vi "trancon-main.vi"() -> ()   [LabVIEW 2015]
uses:
  controls/mylistbox.ctl
  controls/radiobuttons-detection.ctl
  controls/radiobuttons-exp.ctl
  controls/graph.ctl
  dependecies/Error Code Enum typedef.ctl
  controls/clustercontrols-measerument.ctl
  Classes/Experiment.lvclass
  <vilib>/DAQmx/write.llb/DAQmx Write (Digital Bool 1Line 1Point).vi
  <vilib>/DAQmx/read.llb/DAQmx Read (Analog 1D DBL 1Chan NSamp).vi
  <vilib>/Analysis/baseanly.llb/Mean (DBL).vi
  <vilib>/DAQmx/read.llb/DAQmx Read (Digital Bool 1Line 1Point).vi
  dependecies/globalVarSD.vi
  <vilib>/DAQmx/miscellaneous.llb/DAQmx Fill In Error Info.vi
  Classes/Experiments_group.lvclass
  <vilib>/Analysis/NI_AALBase.lvlib
panel:
  in  "Relay key":bool
  in  "Statistics":bool
  in  "shift":i32
  in  "Old/New":bool
  in  "Cut On/off":bool
  in  "pixel-":i32=50
  in  "pixel+":i32=450
  out "moved":string
  in  "Delay (mm) 2":i32 min=-700 max=100
  out "Delay (mm)":dbl
  out "Delay (ps)":dbl=-0.0
  in  "type of movement":u16(ring)=2 items=["definir position", "deplacer relatif", "deplacer absolu"]
  out "deplacement boolean":bool
  in  "Move delay line":bool
  out "Initialisation finie":bool
  in  "STOP":bool
  in  "Work/Dev":bool=TRUE
  in  "Experiment type":T1
  in  "Detection type":T2=enum."UV-vis detection"
  in  "Block accelerator":bool=TRUE
  in  "Block laser beam":bool=TRUE
  in  "Move target":bool
  in  "cellule":u16(ring)=1 items=["Cell1", "Cell2", "Cell stat", "Cell3", "Cell4", "Lanex"]
  out "Cell in place":bool
  in  "Slide":i32(slide)=2 scale=0.0..5.0
  in  "Base path":path=path "G:/SD/DATA"
  out "ALARM":bool
  in  "MainTab":enum32{"Real time", "Measurement", "Settings"}(tab)
  in  "Save SC":bool
  in  "# par point":i32=10 min=1 max=100 step=1
  in  "Real time":bool
  in  "Time, ms":dbl=10.0 min=1.0 max=150.0
  in  "Move Crystall":bool
  out "Réglage TR SC":cluster{"Y":dbl[], "Y":dbl[]}[](graph)=[{"Y"=array[512 elements], "Y"=array[512 elements]}, {"Y"=array[512 elements], "Y"=[6.8, 6.2, 16.4, 11.8, 0.8, 9.8, 11.4, 13.6, 13.0, 10.6, 14.2, 8.6, 15.8, 11.0, 8.6, 12.6, 9.6, 9.4, 16.2, 10.8, 15.6, 11.4, 8.8, 13.6, 10.0, 8.2, 14.8, 17.4, 12.8, 13.2, 18.2, 11.8, 12.8, 17.4, 14.8, 19.4, 21.8, 26.4, 26.6, 35.4, 41.6, 41.0, 55.6, 60.6, 73.0, 85.8, 88.0, 106.6, 125.0, 140.0, 168.6, 188.2, 209.0, 235.2, 267.4, 292.2, 320.8, 351.4, 397.6, 431.8, 475.6, 521.0, 576.2, 623.4, 695.8, 752.0, 833.4, 903.2, 1007.2, 1082.6, 1193.2, 1304.0, 1415.6, 1527.0, 1680.0, 1805.8, 1954.8, 2073.4, 2241.6, 2394.8, 2581.2, 2714.2, 2872.8, 3013.0, 3213.8, 3372.8, 3558.2, 3709.8, 3899.4, 4049.0, 4210.8, 4323.8, 4455.6, 4530.8, 4649.8, 4744.0, 4794.6, 4841.8, 4903.0, 4937.2, 4955.8, 4944.6, 5001.2, 5011.4, 4971.0, 4967.4, 4940.8, 4908.2, 4897.6, 4815.8, 4755.8, 4671.6, 4553.6, 4440.2, 4394.8, 4223.6, 4120.6, 3977.6, 3895.6, 3809.4, 3721.6, 3619.8, 3558.4, 3527.6, 3463.8, 3348.6, 3322.4, 3214.2, 3202.0, 3114.2, 3081.6, 3028.0, 2942.6, 2856.0, 2795.8, 2690.2, 2625.4, 2535.4, 2475.2, 2386.8, 2354.8, 2281.4, 2260.0, 2195.0, 2173.0, 2124.6, 2136.8, 2111.2, 2133.2, 2114.2, 2129.8, 2116.8, 2125.0, 2109.8, 2128.6, 2121.6, 2119.8, 2121.2, 2122.4, 2093.8, 2053.0, 1998.8, 1993.8, 1951.4, 1922.2, 1874.6, 1854.2, 1819.4, 1814.0, 1789.8, 1818.2, 1826.6, 1872.8, 1897.4, 2010.0, 2048.2, 2125.8, 2138.2, 2201.8, 2220.2, 2249.8, 2255.6, 2238.8, 2188.8, 2164.8, 2103.4, 2020.4, 1918.8, 1836.0, 1712.0, 1602.4, 1516.4, 1454.8, 1355.2, 1259.0, 1217.8, 1176.2, 1109.6, 1119.4, 1105.2, 1125.6, 1167.2, 1260.4, 1364.4, 1490.8, 1615.0, 1791.8, 1904.0, 2039.4, 2136.6, 2245.0, 2243.6, 2354.2, 2386.6, 2434.0, 2424.0, 2440.2, 2390.0, 2371.8, 2304.0, 2249.2, 2138.0, 2070.4, 1940.8, 1837.6, 1741.6, 1637.4, 1525.2, 1440.2, 1337.4, 1259.6, 1161.8, 1088.6, 1018.8, 954.0, 895.0, 853.2, 793.6, 761.8, 714.4, 693.0, 644.2, 621.8, 580.4, 565.4, 540.6, 521.2, 499.0, 488.4, 464.2, 453.6, 433.0, 425.2, 413.0, 414.4, 391.6, 388.6, 366.0, 368.0, 342.2, 337.4, 316.2, 303.6, 290.2, 278.4, 267.8, 258.4, 241.8, 240.0, 220.2, 221.4, 192.2, 187.2, 167.6, 154.6, 144.6, 137.8, 131.2, 123.4, 107.2, 114.4, 98.0, 98.8, 88.0, 81.0, 75.6, 82.8, 78.0, 72.0, 65.2, 67.4, 62.4, 65.2, 62.0, 60.0, 52.6, 50.2, 47.6, 49.4, 40.6, 45.4, 40.8, 47.4, 41.2, 49.6, 39.0, 42.4, 32.4, 33.4, 32.8, 32.6, 32.4, 35.2, 33.8, 33.8, 33.2, 34.4, 29.2, 33.0, 31.0, 35.4, 28.2, 30.4, 32.6, 27.4, 29.0, 33.8, 33.0, 38.6, 30.0, 34.2, 31.8, 40.0, 33.8, 38.4, 32.0, 38.0, 34.0, 38.4, 31.8, 33.2, 30.6, 34.8, 34.2, 34.8, 25.6, 33.6, 27.8, 36.8, 31.4, 31.2, 28.2, 36.2, 30.6, 27.2, 29.2, 18.0, 20.6, 25.2, 25.2, 21.0, 24.8, 27.0, 23.8, 28.8, 16.2, 26.4, 18.8, 21.8, 16.4, 14.8, 12.0, 18.0, 20.8, 18.2, 10.4, 18.8, 18.4, 15.8, 17.8, 19.2, 16.6, 13.8, 13.4, 16.0, 16.8, 18.2, 15.2, 13.4, 13.8, 16.4, 12.2, 16.0, 14.2, 16.4, 12.2, 21.4, 10.8, 20.0, 12.4, 19.0, 13.8, 23.2, 12.8, 10.2, 12.0, 8.4, 8.6, 19.0, 11.6, 28.4, 11.8, 12.8, 13.8, 14.4, 10.8, 12.0, 6.6, 12.2, 11.2, 18.0, 15.4, 21.8, 10.2, 15.2, 10.4, 10.6, 5.0, 8.6, 7.6, 9.8, 7.4, 13.2, 10.6, 15.2, 7.8, 13.4, 12.6, 15.8, 11.6, 12.6, 9.6, 12.6, 12.2, 15.8, 6.2, 14.2, 12.8, 15.6, 7.0, 12.0, 12.8, 15.8, 10.4, 16.2, 11.6, 18.2, 13.0, 12.8, 6.2, 21.4, 9.2, 11.6, 6.0, 8.0, 6.0, 10.6, 6.0, 14.4, 4.8, 10.4, 9.0, 14.0, 11.0, 11.6, 9.2, 11.4, 4.2, 7.2, 5.8, 11.2, 8.2, 11.0, 8.0, 10.2, 5.6, 9.6, 3.6, 12.2, 6.4, 8.2, 4.2, 4.2, 4.0, 2.6, 9.0, 7.0, 5.6, 8.0, 4.6, 11.2, 4.8, 7.8, 3.4, 6.8, 6.8, 9.2, 7.4, 0.4, 5.0, -1.2, 0.0]}, {"Y"=array[512 elements], "Y"=array[512 elements]}, {"Y"=array[512 elements], "Y"=array[512 elements]}]
  out "Réglage TR OD":T3(graph)
  in  "wavelength fix":dbl=640.0 caption="wave fix"
  in  "ODmax":dbl=1.0
  in  "ODmin":dbl=-1.0
  in  "# par point":i32=15 min=1 max=100 step=1
  out "# current":i32
  out "RDT, ps":dbl=3790.0
  out "Real time exp":T4
  in  "sigma":dbl=1.4 min=0.0 step=0.1
  in  "Clean":bool
  in  "load Exp":bool
  in  "BG correct":bool
  in  "Save":bool
  in  "del exp":bool
  in  "del group":bool
  in  "add exp":bool
  in  "add group":bool
  in  "All":bool
  in  "Average exp":bool
  in  "clean mode":enum32{"delete", "approximate"}(radio)=enum."approximate"
  in  "Commentaires exp":string="...Write experiment description..."
  in  "Commentaires group":string="...write group description..."
  in  "Experiment":T5
  in  "group":u16(ring) items=["1. Init exp", "2. 120417"]
  in  "LogY":bool
  in  "sel kin":i32
  in  "Avr kinetics":bool
  in  "Del kinetics":bool
  in  "Add kinetics":bool
  in  "To Wave":dbl
  in  "From Wave":dbl
  out "Kinetics":cluster{"Y":dbl[], "Y":dbl[]}[](graph)
  in  "DelaysTab":enum32{"Mode Normale", "Table"}(tab)
  in  "Fix":bool=TRUE
  in  "Break measurement":bool
  in  "# points":i32=1 min=1 step=1
  in  "OZ, ps":dbl=-250.0 min=-1000.0 max=9000.0
  in  "step, ps":dbl=15.0 min=-100.0 max=1000.0 step=1.0
  out "Total, ps":dbl=3990.0
  out "Kinetics, ps":dbl=3790.0 min=-200.0 max=8350.0
  in  "load table":bool
  in  "Table path":path=path "C:/Users/Sergey Denisov/Dropbox/LCP/Soft/LabVIEW/TRANCON-2016/delay/main-delay.txt"
  in  "sel. wavelen.":dbl[](array[numeric])=[370.0, 400.0, 450.0, 500.0, 550.0, 600.0, 640.0, 700.0]
  out "Accelerator":bool
  in  "Start measurement":bool
  in  "Log":bool
  in  "def pixel-":dbl
  in  "def pixel+":dbl=5.0
  in  "Exp name":string
  in  "Name group":string
  in  "aq contol":enum32{"fixed", "automatic", "fixed-auto"}(radio)
  in  "save Radio Buttons":enum32{"Automatic", "User-def"}(radio)
  out "slider":dbl(slide) scale=0.0..1.0
  out "error":dbl(knob) scale=1e-09..1e-05 scale format="%#_2e"
  in  "error min":dbl=0.001 format="%#_6e"
  in  "sel spect":i32
  in  "Avr spectrum":bool
  in  "Del spectrum":bool
  in  "Add spectrum":bool
  in  "To Time":dbl
  in  "From Time":dbl
  out "Spectrum O.D.":cluster{"Y":dbl[], "Y":dbl[]}[](graph)
  out "GRAPH EXPERIMENTAL DATA":dbl[][](graph)=[[1.0, 1.0], [1.0, 1.0]]
  in  "accuracy":string="%.4f"
  in  "path alarm sound":path=path "G:/SD/TRANCON/sounds/swgzq-rkyg3.wav"
  in  "current Alarm break, uA":dbl=100.0 format="%#_13g"
  in  "current Alarm, uA":dbl=1000.0 format="%#_13g"
  out "Alarm current":dbl
  in  "real Zero":dbl=-10.0
  out "Initialization OK":bool=TRUE
  out "delay":dbl
  out "MaxRange cell":dbl=70.0 format="%.2f"
  out "MinRange cell":dbl=-100.0 format="%.2f"
  out "MaxRange":dbl=100.0 format="%.2f"
  out "MinRange":dbl=-700.0 format="%.2f"
  in  "Pixel test":i32=300
  in  "Seuil SC Ref":dbl=2500.0
  in  "Seuil SC Sig":dbl=2500.0
  out "error out":errorcluster
  in  "pos of targets":dbl[](array[numeric])=[48.0, 24.0, 0.0, -24.0, -48.0, 35.0] min=-70.0 max=70.0
  in  "Detectors":enum32{"UV-vis-camera"}(tab)
  in  "Check T":bool
  in  "temp set":i32=-35
  in  "cooling":bool=TRUE
  out "Thermometer":i32(slide) scale=-50.0..50.0
  out "status cooling process":T6=enum."DRV_TEMPERATURE_NOT_STABILIZED"
  out "var?":enum32{"var"}(tab)
  out "Block":bool
  in  "table delays":dbl[](array[numeric])=[-300.0, -200.0, -100.0, 0.0, 100.0, 200.0]
  out "wavelengths":dbl[](array[numeric])=[1.74695840294851, 1.73947371440581, 1.73199263543554, 1.72451569505241, 1.71704336159476, 1.70957618537218, 1.70211465103603, 1.69465931938089, 1.68721070135242, 1.6797693560201301, 1.67233583286395, 1.66491067290181, 1.65749448123694, 1.65008777499183, 1.64269118936313, 1.63530526816863, 1.62793059787024, 1.62056782564518, 1.6132174869458, 1.60588021624955, 1.59855664914169, 1.59124734594406, 1.58395293766588, 1.57667410341541, 1.56941139768648, 1.56216544706426, 1.55493690232794, 1.54772642715279, 1.54053459790541, 1.53336204673031, 1.5262094059754, 1.5190773076058, 1.51196639712882, 1.50487731519191, 1.49781065537266, 1.49076704050463, 1.48374708968683, 1.4767514175569, 1.4697806335417, 1.46283534108578, 1.45591613685827, 1.44902362355376, 1.4421584350399, 1.43532109764276, 1.42851217454608, 1.42173221797025, 1.41498176826326, 1.40826153129896, 1.40157188671621, 1.39491332390898, 1.38828653993869, 1.38169189429006, 1.37512987969607, 1.36860110805257, 1.3621058521608, 1.35564479016035, 1.3492181722474, 1.34282652069934, 1.33647029749548, 1.33014974492859, 1.32386540164977, 1.31761765329026, 1.31140674343692, 1.30523303537283, 1.29909687508932, 1.29299859208834, 1.28693855623105, 1.28091695705859, 1.27493406221769, 1.26899011878883, 1.26308544991285, 1.25722022338053, 1.25139461273802, 1.2456087796279, 1.23986286216394, 1.23415717021322, 1.22849182981838, 1.2228667403288, 1.2172823138312, 1.21173844101154, 1.20623526099378, 1.20077284844751, 1.19535128728291, 1.18997039739273, 1.18463066565183, 1.17933166025863, 1.174073424022, 1.16885619951437, 1.16367983262934, 1.15854420056361, 1.15344927142328, 1.14839499472779, 1.14338130122296, 1.13840810270664, 1.13347529186764, 1.12858274213783, 1.12373030755832, 1.11891782265939, 1.1141453578523, 1.10941267699039, 1.10471941530734, 1.10006545035942, 1.0954509959156, 1.09087526672658, 1.0863386046025, 1.08184037921328, 1.07738075829889, 1.07295905446028, 1.0685757295472, 1.06422989459505, 1.05992154623097, 1.05565074890564, 1.05141685513876, 1.0472196667672, 1.04305897437087, 1.03893469695662, 1.03484651523027, 1.03079405980805, 1.02677707479348, 1.02279529322078, 1.01884843710765, 1.01493621751393, 1.0110584683138, 1.0072149741535, 1.00340527047478, 0.999629026799409, 0.995885902045937, 0.99217596598108, 0.98849879844413, 0.984853757374839, 0.981241054344726, 0.977660158822735, 0.974110590515482, 0.970592605892286, 0.967105210684661, 0.963648839619437, 0.960222603595605, 0.956826487302473, 0.953460345239886, 0.950123391218081, 0.946815901262915, 0.943537424146781, 0.940287407694674, 0.937065621602715, 0.933872182979098, 0.930706610328418, 0.927568480301523, 0.924457544150809, 0.921373548867979, 0.918316237235768, 0.915285347880829, 0.912280615327582, 0.9093017700531, 0.906348538542966, 0.903420643348089, 0.900517803142482, 0.897639732781836, 0.894786143363061, 0.891956742284595, 0.889151695015634, 0.886370451849697, 0.88361257891826, 0.880877770049898, 0.878166234404625, 0.875477603375355, 0.872811181317668, 0.87016718058367, 0.867545430389945, 0.864945008341113, 0.862366773424345, 0.859809471799701, 0.857273487959592, 0.854758299394799, 0.852263819576187, 0.849789719421444, 0.847335982951904, 0.844901929890081, 0.842488162930783, 0.840093417182113, 0.837718515604053, 0.835362615919645, 0.833025256625637, 0.830707311695789, 0.828407649933811, 0.826126036965772, 0.823862809877985, 0.821617722160325, 0.819390181428017, 0.817180036573831, 0.814987181869723, 0.812812007239723, 0.810653714195849, 0.808512147956872, 0.806387152922779, 0.804278572689575, 0.802186250064211, 0.800110027079448, 0.798049745008728, 0.796005244381085, 0.793976454114127, 0.791963086287712, 0.789964959427523, 0.787981911065323, 0.786013831173131, 0.784060630502893, 0.78212207538586, 0.780198000931301, 0.778288241637713, 0.776392631407606, 0.774511003562155, 0.772643190855895, 0.770789025491363, 0.768948339133666, 0.767121449826945, 0.765307967824209, 0.763507516369203, 0.761719925215525, 0.759945023646196, 0.7581833910296, 0.756434390087585, 0.754697623970222, 0.752972920289276, 0.751261192560027, 0.749561354164361, 0.74787311902268, 0.746197142709487, 0.744533015644908, 0.742880029696423, 0.741239027402037, 0.739609387275517, 0.737990423420732, 0.73638361200569, 0.734787227071191, 0.733201926757378, 0.73162764208114, 0.730063551411954, 0.728510886679627, 0.726967845048158, 0.725436176344851, 0.723913978581447, 0.722402723949191, 0.720900885935728, 0.719409739902714, 0.717927776193409, 0.71645643229521, 0.714993856203966, 0.713542007036553, 0.712098780852969, 0.710665667995441, 0.709241510995812, 0.707826617136283, 0.706421219857516, 0.705024166639125, 0.703637106868306, 0.702258385108918, 0.700888369872632, 0.699527668337694, 0.698175030143386, 0.696831212067962, 0.695496163510531, 0.694169015078566, 0.692850439115762, 0.691540448540173, 0.690238194392353, 0.68894390353484, 0.687658374393696, 0.686380417545913, 0.685109988189973, 0.68384778746451, 0.682593529592659, 0.681346634578122, 0.680107057481696, 0.678875371772439, 0.677651411261084, 0.676434603603688, 0.675224903742191, 0.674022266593929, 0.672827515950317, 0.671639819004719, 0.670459019270995, 0.66928507156971, 0.668117930701417, 0.666957767455301, 0.665804889055705, 0.664658651647345, 0.663519009955227, 0.662385918688791, 0.661259332542666, 0.660139206197413, 0.659025494320265, 0.657918577745861, 0.656818087211363, 0.655723844942282, 0.654635805560979, 0.653553923680618, 0.652478153905886, 0.651408450833686, 0.65034476905383, 0.649287063149737, 0.648235287699102, 0.647189397274565, 0.6461493464444, 0.645115089773149, 0.644086581822294, 0.643063777150895, 0.642046630316235, 0.641035095874451, 0.640029128381159, 0.639028682392086, 0.63803371246365, 0.6370441731536, 0.636060019021599, 0.635081204629804, 0.634107684543462, 0.633139413331478, 0.632176345566988, 0.631218435827905, 0.630265638697489, 0.629317908764871, 0.628375200625596, 0.627437468882152, 0.626504668144487, 0.625576753030516, 0.624653678166628, 0.623735398188169, 0.622821867739936, 0.621913041476642, 0.62100892535674, 0.620109953829607, 0.61921558033413, 0.618325759554615, 0.617440446187314, 0.616559594940844, 0.61568316053661, 0.614811097709209, 0.613943361206831, 0.613080378184452, 0.612221994630098, 0.611367831427453, 0.610517843366502, 0.60967198525252, 0.60883021190643, 0.60799247816513, 0.607159693604442, 0.60633093309446, 0.605506106395553, 0.604685168394393, 0.603868073995068, 0.60305511142711, 0.602246732258074, 0.601442091036539, 0.6006411427212, 0.599843842289426, 0.599050453455946, 0.598261610552242, 0.597476310031922, 0.596694506931211, 0.595916156306054, 0.595142093000695, 0.594371942537607, 0.593605139217181, 0.592841638157853, 0.592081906172738, 0.591326408617177, 0.590574108124154, 0.58982495987703, 0.589079419713967, 0.588338078537831, 0.587599784549585, 0.586864492999568, 0.586133005237403, 0.585405324564155, 0.584680541417083, 0.583958611115143, 0.5832410364252, 0.582526521056125, 0.581814753770653, 0.581106377109973, 0.58040188911896, 0.579700044555559, 0.579000804083577, 0.578306103301326, 0.577613941398089, 0.576924273860396, 0.576238621805796, 0.575555902738057, 0.574875573645619, 0.574198903353956, 0.573525387538455, 0.572854157418386, 0.572186407197363, 0.571521855295781, 0.570859484920937, 0.570200593127219, 0.569544766049075, 0.56889101644063, 0.56824092148275, 0.567593580387639, 0.566948212816984, 0.566306853158223, 0.565667759457371, 0.565030744389789, 0.564397849608573, 0.563766764965671, 0.563138393001049, 0.562513372853575, 0.561890059184882, 0.561270268935877, 0.560652885480491, 0.560037363089153, 0.559425835098158, 0.558815850645196, 0.558208818010672, 0.557604554961745, 0.557001744243597, 0.55640312797365, 0.555805892569102, 0.555211479804027, 0.554619757339678, 0.554029520629567, 0.553443236604538, 0.552858171035084, 0.552276240638747, 0.551696479889713, 0.551118679771488, 0.550544149465713, 0.549970675460912, 0.549401090190914, 0.548832713227076, 0.548267212547523, 0.547703858369913, 0.547142427072201, 0.546584021469991, 0.5460266443561, 0.545473113162201, 0.544920358432839, 0.544371044135748, 0.543823030776167, 0.543277725134077, 0.542734379095834, 0.542193066954772, 0.541654314231999, 0.541116980449427, 0.540582747078486, 0.54004937652346, 0.539519588582563, 0.538990239190229, 0.538464749744689, 0.53793971315779, 0.537418141618218, 0.53689734402556, 0.53637967530906, 0.53586304293919, 0.535349261975299, 0.534836721095929, 0.534326812826771, 0.533818289744137, 0.533312239124593, 0.532807660182776, 0.532305452180648, 0.531804743760851, 0.531306363357019, 0.530809451876789, 0.530314884065384, 0.529821695977794, 0.529330925766354, 0.528841387559125, 0.528354399968765, 0.527868438163348, 0.527385218228913, 0.526902759379507, 0.526423292149745, 0.525944262842272, 0.525468533379988, 0.524992860231003, 0.524520853613227, 0.52404884699545, 0.52358016458692, 0.523111865905063, 0.522646378081368, 0.522181772441391, 0.521719405918609, 0.521258478441176, 0.52079915996126, 0.520341895781911, 0.519885552111302, 0.519431936380601, 0.518978494308777, 0.518528512192482, 0.518078530076188, 0.517631535209674, 0.517185171888899, 0.516740917459748, 0.516298158131117, 0.51585657100424, 0.515417400880057, 0.514978407937087, 0.514542812245489, 0.514107216553891, 0.513674304368112, 0.513242268353238, 0.512811789417832, 0.512383298339977, 0.511955179591973, 0.511530218727756, 0.511105257863537, 0.510682941755925, 0.510261496398444, 0.509841379687589, 0.509423435146592, 0.509005490605594, 0.508590986409599] caption="toutes les lignes" format="%0.3f"
  in  "mimic main cursor move":bool
  in  "Upload wavelength":bool
  in  "Adress wavelength array":path=path "G:/Data/étalonnage/calibration140324.DAT"
  # "OFF"
  # "ON"
  # "all?"
  # "Log"
  # "Ligne à retard"
  # "Paramètres développement"
  # "ON"
  # "OFF"
types:
  T1 = typedef "radiobuttons-exp.ctl" = enum32{"Pump-probe", "Pump-push-probe"}
  T2 = typedef "radiobuttons-detection.ctl" = enum32{"IR detection", "UV-vis detection"}
  T3 = cluster{"wavelengths":dbl[], "TRABS shifted":dbl[]}[]
  T4 = typedef "graph.ctl" = cluster{"wavelengths":dbl[], "OD averaged":dbl[]}[]
  T5 = typedef "mylistbox.ctl" = i32[]
  T6 = typedef "Error Code Enum typedef.ctl" = enum32{"N/A (0)", "DRV_ERROR_CODES", "DRV_SUCCESS", "DRV_VXDNOTINSTALLED", "DRV_ERROR_SCAN", "DRV_ERROR_CHECK_SUM", "DRV_ERROR_FILELOAD", "DRV_UNKNOWN_FUNC", "DRV_ERROR_VXD_INIT", "DRV_ERROR_ADDRESS", "DRV_ERROR_PAGELOCK", "DRV_ERROR_PAGEUNLOCK", "DRV_ERROR_BOARDTEST", "DRV_ERROR_ACK", "DRV_ERROR_UP_FIFO", "DRV_ERROR_PATTERN", "N/A (16)", "DRV_ACQUISITION_ERRORS", "DRV_ACQ_BUFFER", "DRV_ACQ_DOWNFIFO_FULL", "DRV_PROC_UNKONWN_INSTRUCTION", "DRV_ILLEGAL_OP_CODE", "DRV_KINETIC_TIME_NOT_MET", "DRV_ACCUM_TIME_NOT_MET", "DRV_NO_NEW_DATA", "N/A (25)", "DRV_SPOOLERROR", "N/A (27)", "N/A (28)", "N/A (29)", "N/A (30)", "N/A (31)", "N/A (32)", "DRV_TEMPERATURE_CODES", "DRV_TEMPERATURE_OFF", "DRV_TEMPERATURE_NOT_STABILIZED", "DRV_TEMPERATURE_STABILIZED", "DRV_TEMPERATURE_NOT_REACHED", "DRV_TEMPERATURE_OUT_RANGE", "DRV_TEMPERATURE_NOT_SUPPORTED", "DRV_TEMPERATURE_DRIFT", "N/A (41)", "N/A (42)", "N/A (43)", "N/A (44)", "N/A (45)", "N/A (46)", "N/A (47)", "N/A (48)", "DRV_GENERAL_ERRORS", "DRV_INVALID_AUX", "DRV_COF_NOTLOADED", "DRV_FPGAPROG", "DRV_FLEXERROR", "DRV_GPIBERROR", "N/A (55)", "N/A (56)", "N/A (57)", "N/A (58)", "N/A (59)", "N/A (60)", "N/A (61)", "N/A (62)", "N/A (63)", "DRV_DATATYPE", "DRV_DRIVER_ERRORS", "DRV_P1INVALID", "DRV_P2INVALID", "DRV_P3INVALID", "DRV_P4INVALID", "DRV_INIERROR", "DRV_COFERROR", "DRV_ACQUIRING", "DRV_IDLE", "DRV_TEMPCYCLE", "DRV_NOT_INITIALIZED", "DRV_P5INVALID", "DRV_P6INVALID", "DRV_INVALID_MODE", "DRV_INVALID_FILTER", "DRV_I2CERRORS", "DRV_I2CDEVNOTFOUND", "DRV_I2CTIMEOUT", "DRV_P7INVALID", "N/A (84)", "N/A (85)", "N/A (86)", "N/A (87)", "N/A (88)", "N/A (89)", "DRV_IOCERROR", "DRV_VRMVERSIONERROR"}
  T7 = enum8{"Enabled", "Disabled", "Disabled and Grayed Out"}
  T8 = typedef "clustercontrols-measerument.ctl" = cluster{"error":refnum<vi>, "RT exp":refnum<vi>, "# current":refnum<vi>, "Start measurement":refnum<vi>, "GRAPH EXPERIMENTAL DATA":refnum<vi>, "DelaysTab":enum32{"Mode Normale", "Table"}, "slider":refnum<vi>, "aq contol":enum32{"fixed", "automatic", "fixed-auto"}, "RDT, ps":refnum<vi>, "table delays":dbl[], "notifier mesure in":refnum<notifier>, "Measure finished":refnum<user-event>, "Measure event":refnum<user-event>, "Laser shutter task":refnum<k21>, "minmaxOD":cluster{"ODmin":dbl, "ODmax":dbl}}
  T9 = cluster{"Fix":bool, "DeltaT":dbl, "#points":i32, "Delay":dbl}
  T10 = cluster{"Full/Part":bool, "Item names":string[], "Exp number":i32}
  T11 = cluster{"From Time":dbl, "To Time":dbl, "From Wave":dbl, "To Wave":dbl}
  T12 = cluster{"Commentaires exp":refnum<vi>, "GRAPH EXPERIMENTAL DATA":refnum<vi>, "Experiment":refnum<vi>}
  T13 = typedef "control-cluster.ctl" = cluster{"Kinetics":cluster{"timedelay":dbl[], dbl[]}[], "Spectrum":cluster{"Unités abscisse":dbl[], dbl[]}[], "Experiments groups":refnum<class "Experiments_group.lvclass">[], "GRAPH EXPERIMENTAL DATA":dbl[][], "error out":errorcluster, "group":i32, "exp selected":i32, "# exp":i32, "kinetics plot names":string[], "spectra plot names":string[], "FromToWave":cluster{"FromWave":dbl, "ToWave":dbl}, "Laser shutter task":refnum<k21>, "Accelerator task":refnum<k21>, "Motor task":refnum<k21>, "GRAPH EXPERIMENTAL DATA ref":refnum<vi>, "timedelays":dbl[], "wavelengths":dbl[], "Experiment":refnum<vi>, "Commentaires exp":refnum<vi>, "FromToDelay":cluster{"FromDelay":dbl, "ToDelay":dbl}}
  T14 = typedef "Controls.ctl" = cluster{"Update graphs of exp":refnum<user-event>, "Reglage event":refnum<user-event>, "Stop event":refnum<user-event>, "notifier mesure out":refnum<notifier>, "notifier reglage out":refnum<notifier>, "Measure finished":refnum<user-event>, "control registration ref":refnum<event-registration>, "redraw event":refnum<user-event>, "Measure event":refnum<user-event>, "Mes, Reg, Stop Registration ref":refnum<event-registration>, "Laser shutter task":refnum<k21>, "error out":errorcluster, "Motor task":refnum<k21>, "Accelerator task":refnum<k21>, "Faraday Cup task":refnum<k21>, "Protection":refnum<event-registration>, "heater Alarm task":refnum<k21>, "Relay key task":refnum<k21>}
  T15 = cluster{"Unités abscisse":dbl[], "Sig et ref -BG et BGsig et ref":dbl[]}[]
  T16 = cluster{bool, "String File Names":string[], "exp selected":i32}
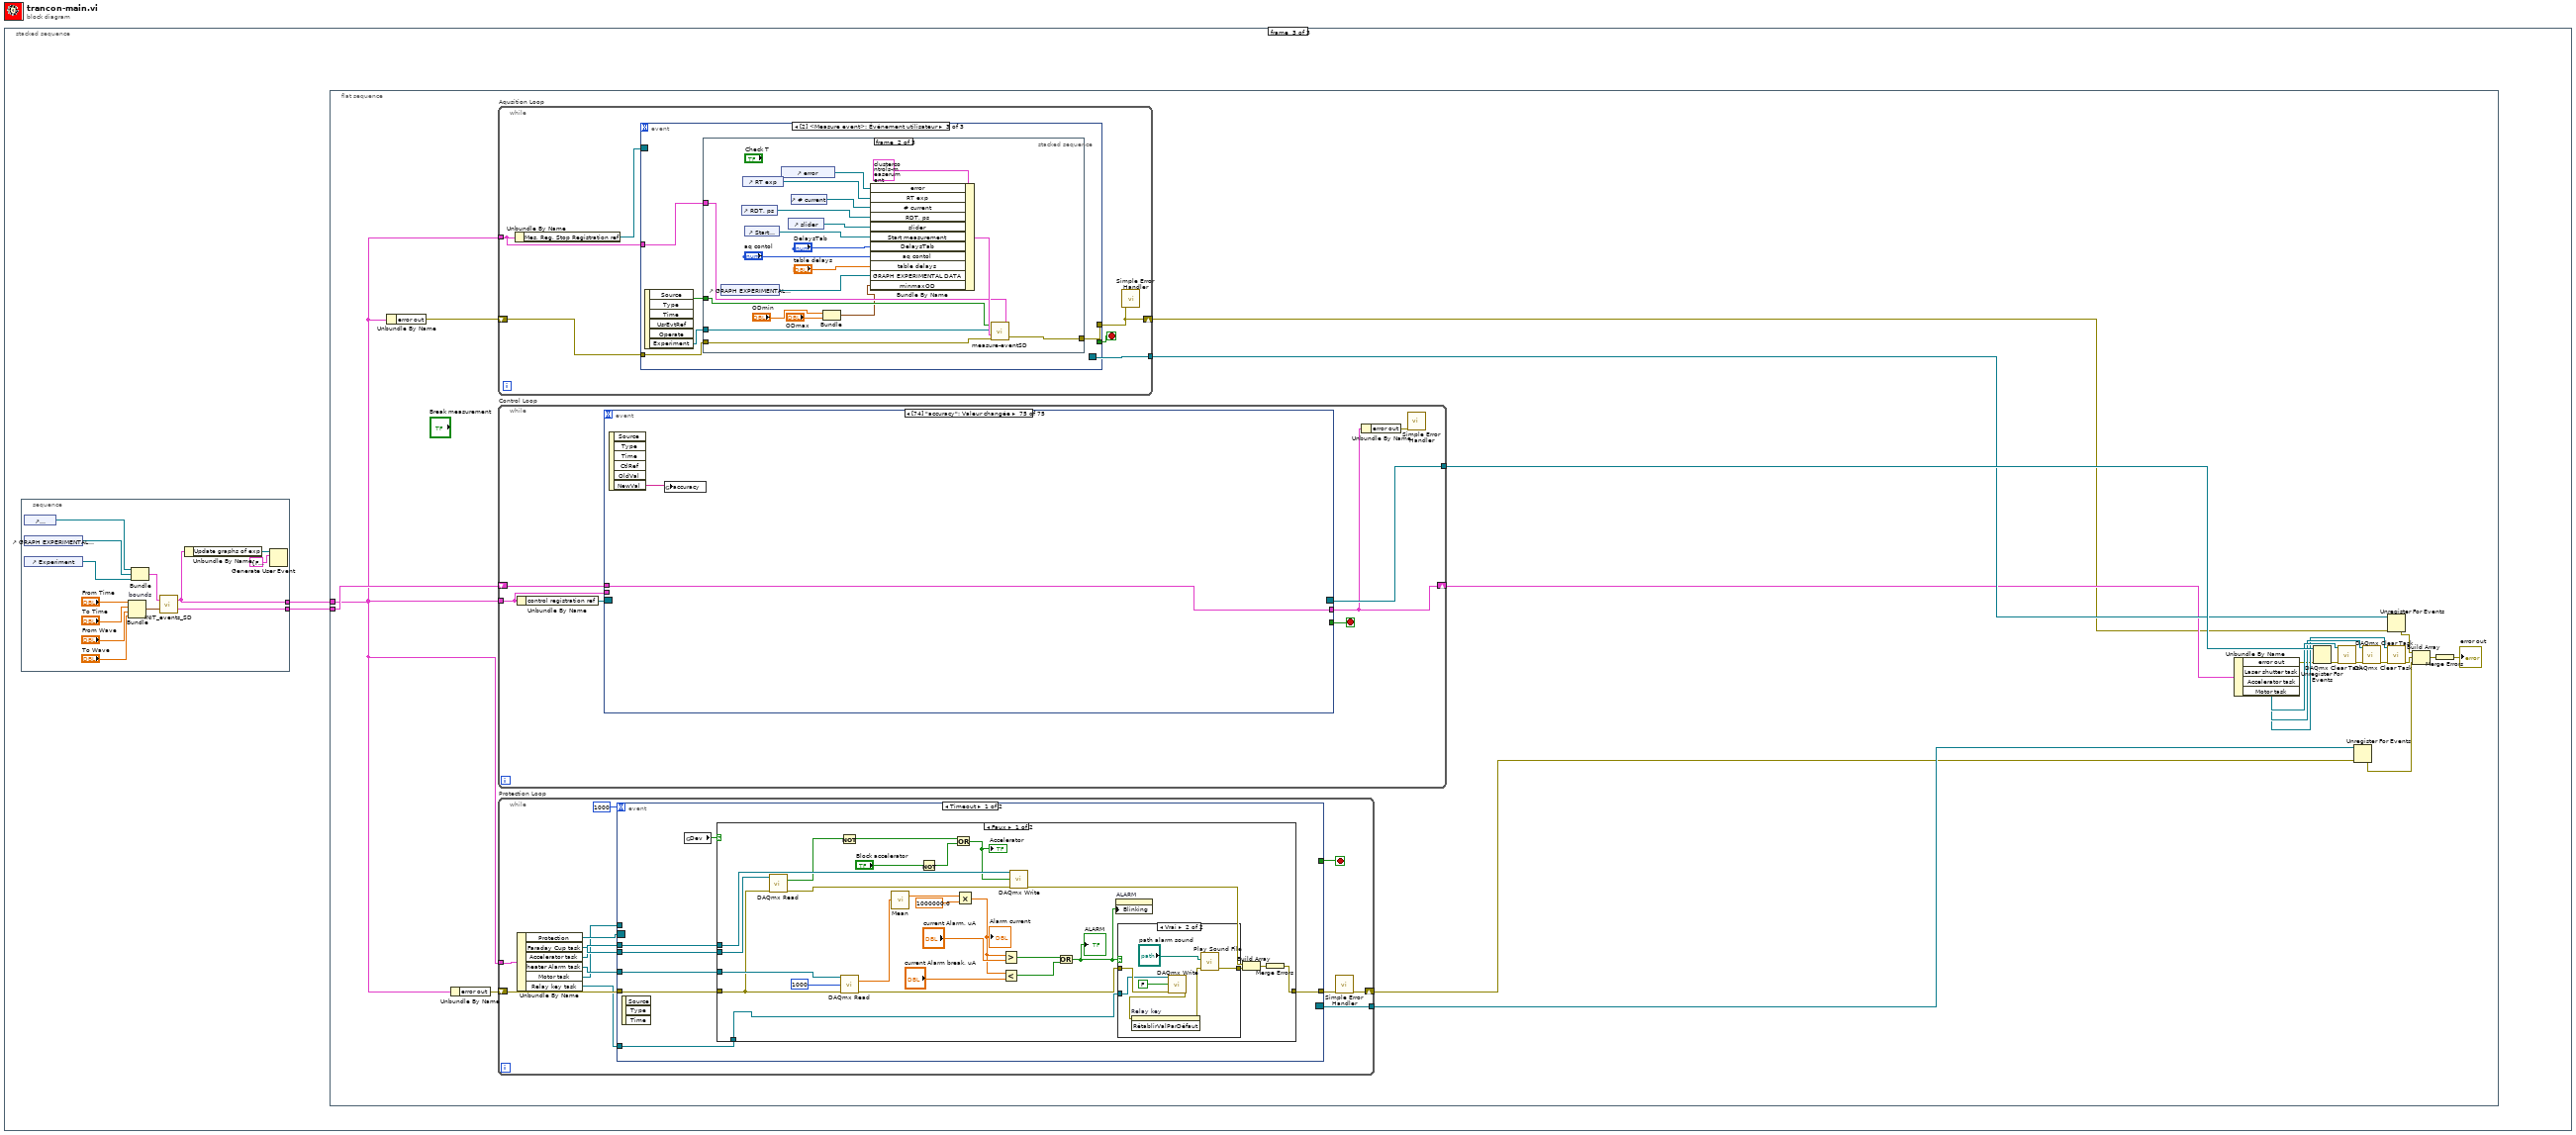
[diagram p0: block diagram]
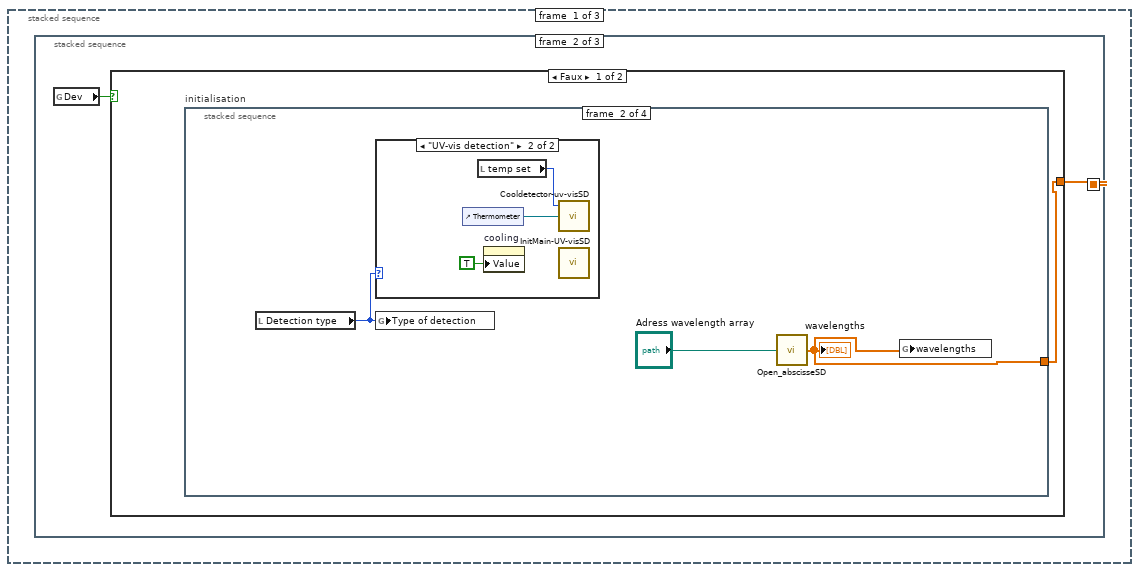
[diagram p2: hidden frame]
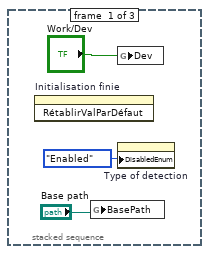
[diagram p3: hidden frame]
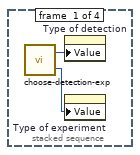
[diagram p4: hidden frame]
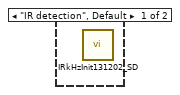
[diagram p5: hidden frame]
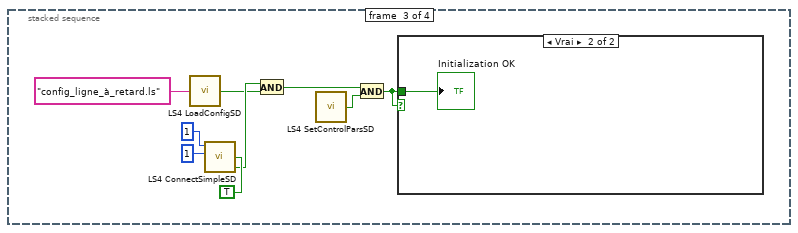
[diagram p6: hidden frame]
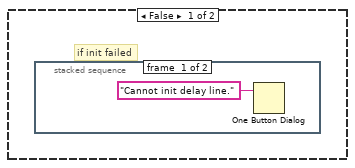
[diagram p7: hidden frame]
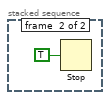
[diagram p8: hidden frame]
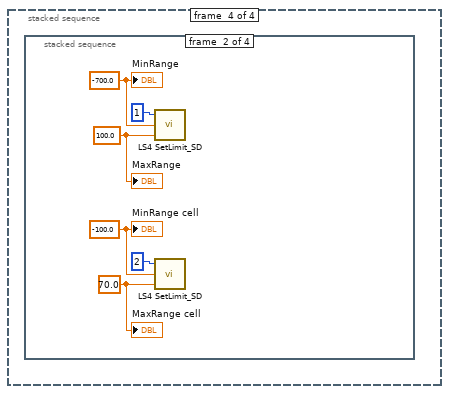
[diagram p9: hidden frame]
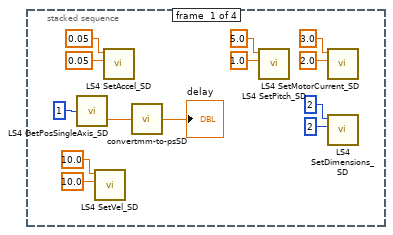
[diagram p10: hidden frame]
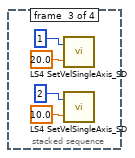
[diagram p11: hidden frame]
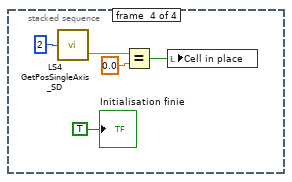
[diagram p12: hidden frame]
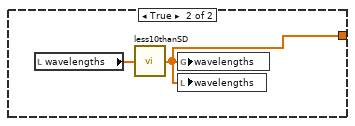
[diagram p13: hidden frame]
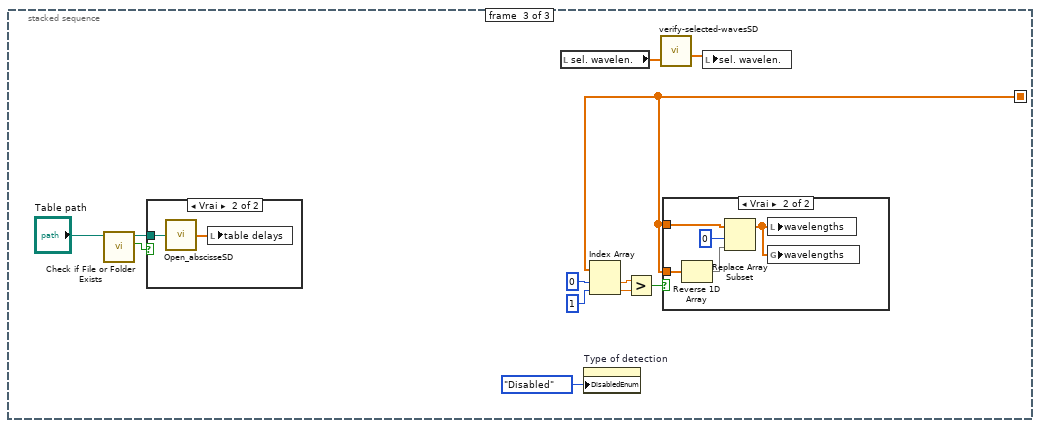
[diagram p14: hidden frame]
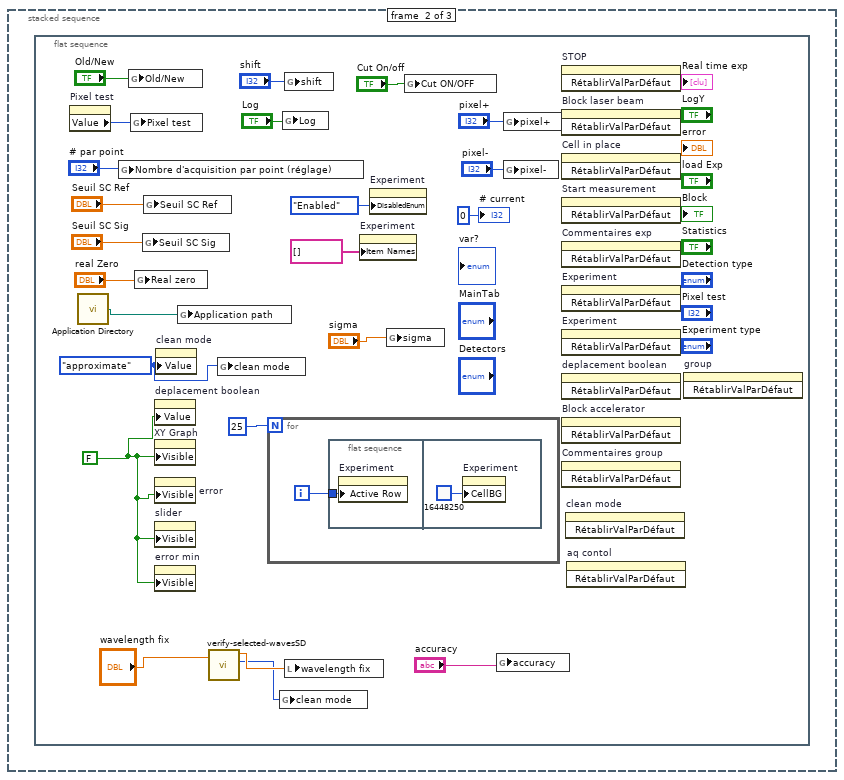
[diagram p17: hidden frame]
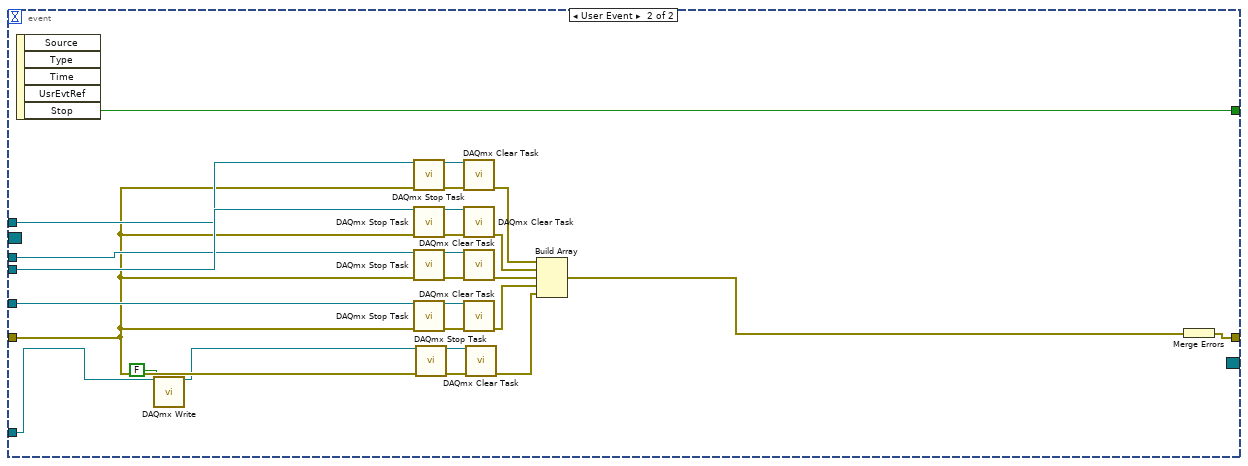
[diagram p20: hidden frame]
diagram:
  n1 = stacked-sequence {
    frame #0 {
      n2 = stacked-sequence {
        seq-local: [_ w4 _] -> [_ _ w58]
        frame #0 {
          n3 = invoke on="Initialisation finie" class="Bool (strict)" method="RétablirValParDéfaut"() -> ()  [unwired: 3 in, 3 out]
          n4 = global write "globalVarSD.vi" "BasePath"("Base path") -> ()
          n5 = global write "globalVarSD.vi" "Dev"("Work/Dev") -> ()
          n6 = property on="Type of detection" class="CmdeBtnsRadio (strict)"("DisabledEnum"=T7."Enabled" ("Disabled")) -> ()  [unwired: 2 in, 2 out]
        }
        frame #1 {
          n7 = global read "globalVarSD.vi" "Dev"() -> (w5:bool)
          n8 = case shown="Faux" w5 {
            tunnel: [w6 w55] -> w4
            frame False {
              n9 = stacked-sequence "initialisation" {
                tunnel: [_ w9 _ _] -> w6
                frame #0 {
                  n10 = call "choose-detection-exp.vi"() -> ("Type of experiment out"=w7:enum32{"Pump-probe", "Pump-push-probe"}, "Type of detection out"=w8:enum32{"IR detection", "UV-vis detection"})  [unwired: 3 in]
                  n11 = property on="Type of detection" class="CmdeBtnsRadio (strict)"("Value"=w8) -> ()  [unwired: 2 in, 2 out]
                  n12 = property on="Type of experiment" class="CmdeBtnsRadio (strict)"("Value"=w7) -> ()  [unwired: 2 in, 2 out]
                }
                frame #1 {
                  n13 = local read "Detection type"() -> (w10:T2)
                  n14 = case shown="\"UV-vis detection\"" w10 {
                    frame "IR detection", Default {
                      n15 = call "IRkHzInit131202_SD.vi"() -> ()  [unwired: 1 in]
                    }
                    frame "UV-vis detection" {
                      n16 = control-ref of="Thermometer"() -> (w13:refnum<vi>)
                      n17 = local read "temp set"() -> (w14:i32)
                      n18 = property on="cooling" class="Bool (strict)"("Value"=TRUE ("cooling")) -> ()  [unwired: 2 in, 2 out]
                      n19 = call "Cooldetector-uv-visSD.vi"("Thermometer"=w13, "temp set"=w14) -> ()  [unwired: 1 in, 2 out]
                      n20 = call "InitMain-UV-visSD.vi"() -> ()  [unwired: 1 out]
                    }
                  }
                  n21 = global write "globalVarSD.vi" "Type of detection"(w10) -> ()
                  n22 = call "Open_abscisseSD.vi"("wavelengts path"="Adress wavelength array") -> ("wavelengths"=w9:dbl[])
                  "wavelengths" <- w9
                  n23 = global write "globalVarSD.vi" "wavelengths"(w9) -> ()
                }
                frame #2 {
                  n24 = call "LS4 LoadConfigSD.vi"("FileName"="config_ligne_à_retard.ls") -> ("Command executed"=w19:bool)
                  n25 = call "LS4 ConnectSimpleSD.vi"("Show Protocol"=TRUE, "COM Port"=u32 1, "Interface (1: RS232; 2: ArcNet; 3: DPRAM)"=u32 1) -> ("Initialization OK"=w20:bool)  [unwired: 3 in]
                  n26 = And(x=w20, y=w19) -> (x .and. y?=w18:bool)
                  n27 = call "LS4 SetControlParsSD.vi"() -> ("Command executed"=w17:bool)
                  n28 = And(x=w18, y=w17) -> (x .and. y?=w15:bool)
                  n29 = case shown="Vrai" w15 {
                    tunnel: w15 -> [_ w26]
                    frame False {
                      # "if init failed"
                      n30 = stacked-sequence {
                        frame #0 {
                          n31 = One Button Dialog(message="Cannot init delay line.") -> ()  [unwired: 1 in, 1 out]
                        }
                        frame #1 {
                          n32 = Stop(stop? (T)=TRUE) -> ()
                        }
                      }
                    }
                    frame True {
                      "Initialization OK" <- w26
                    }
                  }
                }
                frame #3 {
                  n33 = stacked-sequence {
                    frame #0 {
                      n34 = call "LS4 GetPosSingleAxis_SD.vi"("Axis"=1) -> ("Pos"=w30:dbl)  [unwired: 1 out]
                      n35 = call "LS4 SetVel_SD.vi"("Y"=10.0, "X"=10.0) -> ()  [unwired: 2 in, 1 out]
                      n36 = call "LS4 SetAccel_SD.vi"("Y"=0.05, "X"=0.05) -> ()  [unwired: 2 in, 1 out]
                      n37 = call "convertmm-to-psSD.vi"("mm"=w30) -> ("ps"=→"delay":dbl)
                      n38 = call "LS4 SetPitch_SD.vi"("Y"=1.0, "X"=5.0) -> ()  [unwired: 2 in, 1 out]
                      n39 = call "LS4 SetMotorCurrent_SD.vi"("Y"=2.0, "X"=3.0) -> ()  [unwired: 2 in, 1 out]
                      n40 = call "LS4 SetDimensions_SD.vi"("YD"=2, "XD"=2) -> ()  [unwired: 2 in, 1 out]
                    }
                    frame #1 {
                      w40 = 70.0 ("MinRange")
                      w41 = -100.0 ("MinRange")
                      w43 = 100.0 ("MinRange")
                      w44 = -700.0 ("MinRange")
                      n41 = call "LS4 SetLimit_SD.vi"("MaxRange"=w43, "MinRange"=w44, "Axis"=1) -> ()  [unwired: 1 out]
                      n42 = call "LS4 SetLimit_SD.vi"("MaxRange"=w40, "MinRange"=w41, "Axis"=2) -> ()  [unwired: 1 out]
                      "MinRange" <- w44
                      "MaxRange" <- w43
                      "MinRange cell" <- w41
                      "MaxRange cell" <- w40
                    }
                    frame #2 {
                      n43 = call "LS4 SetVelSingleAxis_SD.vi"("Vel"=20.0, "Axis"=1) -> ()  [unwired: 1 out]
                      n44 = call "LS4 SetVelSingleAxis_SD.vi"("Vel"=10.0, "Axis"=2) -> ()  [unwired: 1 out]
                    }
                    frame #3 {
                      n45 = call "LS4 GetPosSingleAxis_SD.vi"("Axis"=2) -> ("Pos"=w52:dbl)  [unwired: 1 out]
                      n46 = Equal?(x=w52, y=0.0) -> (x = y?=w50:bool)
                      n47 = local write "Cell in place"(w50) -> ()
                      "Initialisation finie" <- TRUE
                    }
                  }
                }
              }
            }
            frame True {
              n48 = local read "wavelengths"() -> (w56:dbl[])
              n49 = call "less10thanSD.vi"("Array In"=w56) -> ("Array In out"=w55:dbl[])
              n50 = global write "globalVarSD.vi" "wavelengths"(w55) -> ()
              n51 = local write "wavelengths"(w55) -> ()
            }
          }
        }
        frame #2 {
          n52 = call <vilib>:"Check if File or Folder Exists.vi"("path"="Table path") -> ("file or folder exists?"=w61:bool, "dup path"=w60:path)  [unwired: 8 in, 1 out]
          n53 = case shown="Vrai" w61 {
            tunnel: w60 -> [_ w70]
            frame False {
            }
            frame True {
              n54 = call "Open_abscisseSD.vi"("wavelengts path"=w70) -> ("wavelengths"=w69:dbl[])
              n55 = local write "table delays"(w69) -> ()
            }
          }
          n56 = local read "sel. wavelen."() -> (w57:dbl[])
          n57 = property on="Type of detection" class="CmdeBtnsRadio (strict)"("DisabledEnum"=T7."Disabled" ("Disabled")) -> ()  [unwired: 2 in, 2 out]
          n58 = Index Array(array=w58, index #1=0 ("index"), index #2=1 ("index")) -> (element #1=w66:dbl, element #2=w65:dbl)
          n59 = Greater?(x=w66, y=w65) -> (0:w64:bool)
          n60 = call "verify-selected-wavesSD.vi"("selected wavelengths"=w57) -> ("selected wavelengths out"=w59:dbl[])  [unwired: 1 in, 3 out]
          n61 = case shown="Vrai" w64 {
            tunnel: w58 -> [_ w75]
            tunnel: w58 -> [_ w72]
            frame False {
            }
            frame True {
              n62 = Reverse 1D Array(array=w75) -> (reversed array=w74:dbl[])
              n63 = Replace Array Subset(array=w72, new element=w74, index=0) -> (w71:dbl[])
              n64 = local write "wavelengths"(w71) -> ()
              n65 = global write "globalVarSD.vi" "wavelengths"(w71) -> ()
            }
          }
          n66 = local write "sel. wavelen."(w59) -> ()
        }
      }
    }
    frame #1 {
      n67 = flat-sequence {
        frame #0 {
          w80 = enum32{"delete", "approximate"}."approximate" ("clean mode")
          w82 = FALSE ("Visible")
          n68 = property on="Pixel test" class="NumNb (strict)"() -> ("Value"=w94:i32)  [unwired: 2 in, 2 out]
          n69 = call <vilib>:"Application Directory.vi"() -> ("Application Directory"=w84:path)
          n70 = global write "globalVarSD.vi" "Nombre d'acquisition par point (réglage)"("# par point") -> ()
          n71 = global write "globalVarSD.vi" "Old/New"("Old/New") -> ()
          n72 = global write "globalVarSD.vi" "Pixel test"(w94) -> ()
          n73 = global write "globalVarSD.vi" "Real zero"("real Zero") -> ()
          n74 = global write "globalVarSD.vi" "Seuil SC Sig"("Seuil SC Sig") -> ()
          n75 = global write "globalVarSD.vi" "Seuil SC Ref"("Seuil SC Ref") -> ()
          n76 = property on="deplacement boolean" class="Bool (strict)"("Value"=w82) -> ()  [unwired: 2 in, 2 out]
          n77 = property on="XY Graph" class="GraphXY (strict)"("Visible"=w82) -> ()  [unwired: 2 in, 2 out]
          n78 = property on="error" class="BoutRot (strict)"("Visible"=w82) -> ()  [unwired: 2 in, 2 out]
          n79 = property on="slider" class="Gliss (strict)"("Visible"=w82) -> ()  [unwired: 2 in, 2 out]
          n80 = property on="error min" class="NumNb (strict)"("Visible"=w82) -> ()  [unwired: 2 in, 2 out]
          n81 = property on="clean mode" class="CmdeBtnsRadio (strict)"("Value"=w80) -> ()  [unwired: 2 in, 2 out]
          n82 = global write "globalVarSD.vi" "Application path"(w84) -> ()
          n83 = call "verify-selected-wavesSD.vi"("in wave"="wavelength fix") -> ("closet wave"=w78:dbl, "closest index"=w77:i32)  [unwired: 1 in, 2 out]
          n84 = global write "globalVarSD.vi" "clean mode"(w80) -> ()
          n85 = for {
            N: 25 -> [_]
            i -> [w99]
            n86 = flat-sequence {
              tunnel: w99 -> [w100]
              frame #0 {
                n87 = property on="Experiment" class="LstDér (strict)"("Active Row"=w100) -> ()  [unwired: 2 in, 2 out]
              }
              frame #1 {
                n88 = property on="Experiment" class="LstDér (strict)"("CellBG"=u32 16448250) -> ()  [unwired: 2 in, 2 out]
              }
            }
          }
          n89 = global write "globalVarSD.vi" "clean mode"(w77) -> ()
          n90 = global write "globalVarSD.vi" "Log"("Log") -> ()
          n91 = global write "globalVarSD.vi" "shift"("shift") -> ()
          n92 = local write "wavelength fix"(w78) -> ()
          n93 = property on="Experiment" class="LstDér (strict)"("Item Names"=string[] []) -> ()  [unwired: 2 in, 2 out]
          n94 = property on="Experiment" class="LstDér (strict)"("DisabledEnum"=T7."Enabled" ("Disabled")) -> ()  [unwired: 2 in, 2 out]
          n95 = global write "globalVarSD.vi" "sigma"("sigma") -> ()
          n96 = global write "globalVarSD.vi" "Cut ON/OFF"("Cut On/off") -> ()
          n97 = global write "globalVarSD.vi" "accuracy"("accuracy") -> ()
          n98 = global write "globalVarSD.vi" "pixel+"("pixel+") -> ()
          n99 = global write "globalVarSD.vi" "pixel-"("pixel-") -> ()
          n100 = invoke on="STOP" class="Bool" method="RétablirValParDéfaut"() -> ()  [unwired: 3 in, 3 out]
          n101 = invoke on="Block laser beam" class="Bool (strict)" method="RétablirValParDéfaut"() -> ()  [unwired: 3 in, 3 out]
          n102 = invoke on="Cell in place" class="Bool (strict)" method="RétablirValParDéfaut"() -> ()  [unwired: 3 in, 3 out]
          n103 = invoke on="Start measurement" class="Bool (strict)" method="RétablirValParDéfaut"() -> ()  [unwired: 3 in, 3 out]
          n104 = invoke on="Commentaires exp" class="Str" method="RétablirValParDéfaut"() -> ()  [unwired: 3 in, 3 out]
          n105 = invoke on="Experiment" class="LstBox (strict)" method="RétablirValParDéfaut"() -> ()  [unwired: 3 in, 3 out]
          n106 = invoke on="Experiment" class="LstBox (strict)" method="RétablirValParDéfaut"() -> ()  [unwired: 3 in, 3 out]
          n107 = invoke on="deplacement boolean" class="Bool (strict)" method="RétablirValParDéfaut"() -> ()  [unwired: 3 in, 3 out]
          n108 = invoke on="Block accelerator" class="Bool (strict)" method="RétablirValParDéfaut"() -> ()  [unwired: 3 in, 3 out]
          n109 = invoke on="Commentaires group" class="Str" method="RétablirValParDéfaut"() -> ()  [unwired: 3 in, 3 out]
          n110 = invoke on="clean mode" class="CmdeBtnsRadio (strict)" method="RétablirValParDéfaut"() -> ()  [unwired: 3 in, 3 out]
          n111 = invoke on="aq contol" class="CmdeBtnsRadio (strict)" method="RétablirValParDéfaut"() -> ()  [unwired: 3 in, 3 out]
          n112 = invoke on="group" class="MDér (strict)" method="RétablirValParDéfaut"() -> ()  [unwired: 3 in, 3 out]
          "# current" <- 0 ("# current")
        }
      }
    }
    frame #2 {
      n113 = stacked-sequence {
        tunnel: [w841] -> w102
        tunnel: [w840] -> w103
        frame #0 {
          n114 = control-ref of="Commentaires exp"() -> (w834:refnum<vi>)
          n115 = control-ref of="GRAPH EXPERIMENTAL DATA"() -> (w833:refnum<vi>)
          n116 = control-ref of="Experiment"() -> (w832:refnum<vi>)
          n117 = Bundle "bounds"("From Time"="From Time", "To Time"="To Time", "From Wave"="From Wave", "To Wave"="To Wave") -> (w835:T11)  [unwired: 1 in]
          n118 = Bundle("Commentaires exp"=w834, "GRAPH EXPERIMENTAL DATA"=w833, "Experiment"=w832) -> (w830:T12)  [unwired: 1 in]
          n119 = call "INIT_events_SD.vi"("bounds"=w835, "references"=w830) -> ("main cluster"=w840:T13, "Controls"=w841:T14)
          n120 = Unbundle By Name(w841) -> ("Update graphs of exp"=w829:refnum<user-event>)
          n121 = Generate User Event(user event=w829, event data cluster=T10 {"Full/Part"=FALSE, "Item names"=[], "Exp number"=0} ("Update graphs of exp 2")) -> ()  [unwired: 2 in, 2 out]
        }
      }
      n122 = flat-sequence {
        tunnel: w103 -> [w125]
        tunnel: w102 -> [w104]
        frame #0 {
          n123 = Unbundle By Name(w104) -> ("error out"=w118:errorcluster)
          n124 = Unbundle By Name(w104) -> ("error out"=w117:errorcluster)
          n125 = while "Aqusition Loop" {
            tunnel: [w210] -> w123
            shift-right: [w208] -> w105
            shift-left: w118 -> [w209]
            tunnel: w104 -> [w206]
            stop <- w211 stop-if-true
            n126 = Unbundle By Name(w206) -> ("Mes, Reg, Stop Registration ref"=w207:refnum<event-registration>)
            n127 = event shown="[2] <Measure event>: Événement utilisateur" {
              selector: w207 -> [_ _ _]
              dyn-events: [_ _ _] -> w210
              timeout: _ -> [_ _ _]
              tunnel: [w213 _ _] -> w211
              tunnel: [w212 w215 w236] -> w208
              tunnel: w209 -> [w212 w215 w234]
              tunnel: w206 -> [_ w214 w235]
              event User Event {
                n128 = event-data() -> ("Stop"=w213:bool)  [unwired: 1 in, 4 out]
              }
              event User Event {
                n129 = event-data() -> ("Operate"=w216:bool)  [unwired: 1 in, 4 out]
                n130 = case shown="Vrai" w216 {
                  tunnel: w214 -> [_ w217]
                  frame False {
                  }
                  frame True {
                    n131 = stacked-sequence {
                      tunnel: w217 -> [w222 w225]
                      frame #0 {
                        n132 = Unbundle By Name(w222) -> ("Laser shutter task"=w220:refnum<k21>)
                        n133 = call "reglage-newSD.vi"() -> ("OD"=→"Réglage TR OD":T3, "SC"=→"Réglage TR SC":T15)  [unwired: 1 in]
                        n134 = call-poly <vilib>:"DAQmx Write.vi"("task/channels in"=w220, "data"=TRUE) -> ()  [unwired: 11 in, 3 out]
                      }
                      frame #1 {
                        n135 = Unbundle By Name(w225) -> ("notifier reglage out"=w224:refnum<notifier>)
                        n136 = Get Notifier Status(notifier=w224) -> (current notification=w228:bool)  [unwired: 1 in, 4 out]
                        n137 = case shown="Vrai" w228 {
                          tunnel: [cluster{"Operate":bool} {"Operate"=FALSE} ("event data") cluster{"Operate":bool} {"Operate"=TRUE} ("event data")] -> w229
                          tunnel: [FALSE ("Operate") TRUE ("Operate")] -> w227
                          frame False {
                          }
                          frame True {
                          }
                        }
                        n138 = Unbundle By Name(w225) -> ("Laser shutter task"=w223:refnum<k21>, "Reglage event"=w226:refnum<user-event>)
                        n139 = Generate User Event(user event=w226, event data cluster=w229) -> ()  [unwired: 2 in, 2 out]
                        n140 = call-poly <vilib>:"DAQmx Write.vi"("task/channels in"=w223, "data"=w227) -> ()  [unwired: 11 in, 3 out]
                      }
                    }
                  }
                }
              }
              event User Event {
                n141 = event-data() -> ("Operate"=w238:bool, "Experiment"=w237:refnum<class "Experiment.lvclass">)  [unwired: 1 in, 4 out]
                n142 = stacked-sequence {
                  tunnel: w238 -> [w239 w246 _]
                  tunnel: w237 -> [_ w247 _]
                  tunnel: [_ w259 _] -> w236
                  tunnel: w235 -> [_ w243 _]
                  tunnel: w234 -> [_ w244 _]
                  frame #0 {
                    n143 = property on="XY Graph" class="GraphXY (strict)"("Visible"=w239) -> ()  [unwired: 2 in, 2 out]
                  }
                  frame #1 {
                    n144 = control-ref of="GRAPH EXPERIMENTAL DATA"() -> (w245:refnum<vi>)
                    n145 = control-ref of="RDT, ps"() -> (w254:refnum<vi>)
                    n146 = control-ref of="RT exp"() -> (w251:refnum<vi>)
                    n147 = control-ref of="Start measurement"() -> (w256:refnum<vi>)
                    n148 = control-ref of="error"() -> (w250:refnum<vi>)
                    n149 = control-ref of="slider"() -> (w255:refnum<vi>)
                    n150 = control-ref of="# current"() -> (w252:refnum<vi>)
                    n151 = Bundle("ODmin"="ODmin", "ODmax"="ODmax") -> (w240:cluster{"ODmin":dbl, "ODmax":dbl})  [unwired: 1 in]
                    n152 = Bundle By Name(cluster=T8 {"error"=refnum, "RT exp"=refnum, "# current"=refnum, "Start measurement"=refnum, "GRAPH EXPERIMENTAL DATA"=refnum, "DelaysTab"=enum."Table", "slider"=refnum, "aq contol"=enum."fixed", "RDT, ps"=refnum, "table delays"=[-500.0, -400.0, -0.0, 100.0, 250.0, 350.0], "notifier mesure in"=refnum, "Measure finished"=refnum, "Measure event"=refnum, "Laser shutter task"="", "minmaxOD"={"ODmin"=0.0, "ODmax"=0.0}}, "error"=w250, "RT exp"=w251, "# current"=w252, "RDT, ps"=w254, "slider"=w255, "Start measurement"=w256, "DelaysTab"="DelaysTab", "aq contol"="aq contol", "table delays"="table delays", "GRAPH EXPERIMENTAL DATA"=w245, "minmaxOD"=w240) -> (w248:T8)
                    n153 = call "measure-eventSD.vi"("Controls"=w243, "error in"=w244, "Cluster in"=w248, "Experiment in"=w247, "Operate"=w246) -> ("error out"=w259:errorcluster)
                  }
                  frame #2 {
                    n154 = property on="RDT, ps" class="NumNb (strict)"() -> ("Value"=w263:dbl)  [unwired: 2 in, 2 out]
                    n155 = call "convertps-to-mmSD.vi"("ps"=w263) -> ("mm"=w262:dbl)
                    n156 = Multiply(x=w262, y=-1.0) -> (x*y=w261:dbl)
                    n157 = property on="Delay (ps)" class="NumNb (strict)"("Value"=w263) -> ()  [unwired: 2 in, 2 out]
                    n158 = property on="Delay (mm)" class="NumNb (strict)"("Value"=w261) -> ()  [unwired: 2 in, 2 out]
                  }
                }
              }
            }
            n159 = call <vilib>:"Simple Error Handler.vi"("error in (no error)"=w208) -> ()  [unwired: 4 in, 5 out]
          }
          n160 = while "Control Loop" {
            tunnel: [w269] -> w124
            shift-right: [w267] -> w122
            shift-left: w125 -> [w268]
            tunnel: w104 -> [w264]
            stop <- w270 stop-if-true
            n161 = Unbundle By Name(w264) -> ("control registration ref"=w265:refnum<event-registration>)
            n162 = event shown="[74] \"accuracy\": Valeur changée" {
              selector: w265 -> [_ _ _ _ _ _ _ _ _ _ _ _ _ _ _ _ _ _ _ _ _ _ _ _ _ _ _ _ _ _ _ _ _ _ _ _ _ _ _ _ _ _ _ _ _ _ _ _ _ _ _ _ _ _ _ _ _ _ _ _ _ _ _ _ _ _ _ _ _ _ _ _ _ _ _]
              dyn-events: [_ _ _ _ _ _ _ _ _ _ _ _ _ _ _ _ _ _ _ _ _ _ _ _ _ _ _ _ _ _ _ _ _ _ _ _ _ _ _ _ _ _ _ _ _ _ _ _ _ _ _ _ _ _ _ _ _ _ _ _ _ _ _ _ _ _ _ _ _ _ _ _ _ _ _] -> w269
              timeout: _ -> [_ _ _ _ _ _ _ _ _ _ _ _ _ _ _ _ _ _ _ _ _ _ _ _ _ _ _ _ _ _ _ _ _ _ _ _ _ _ _ _ _ _ _ _ _ _ _ _ _ _ _ _ _ _ _ _ _ _ _ _ _ _ _ _ _ _ _ _ _ _ _ _ _ _ _]
              tunnel: [_ w281 _ _ _ _ _ _ _ _ _ _ _ _ _ _ _ _ _ _ _ _ _ _ _ _ _ _ _ _ _ _ _ _ _ _ _ _ _ _ _ _ _ _ _ _ _ _ _ _ _ _ _ _ _ _ _ _ _ _ _ _ _ _ _ _ _ _ _ _ w799 _ _ _ _] -> w270
              tunnel: w268 -> [w272 w280 w287 w295 w302 w312 w315 w318 w335 w345 w356 w372 w383 w391 w419 w427 w434 w444 w447 w451 w464 w473 w482 w492 w501 w508 w514 w517 w521 w523 w534 w543 w552 w563 w565 w569 w578 w581 w586 w588 w590 w593 w596 w598 w601 w613 w624 w635 w638 w639 w655 w658 w664 w678 w690 w692 w697 w699 w700 w702 w704 w708 w710 w724 w741 w770 w781 w792 w796 w797 w802 w808 w813 w817 w827]
              tunnel: [w272 w280 w287 w295 w302 w312 w315 w319 w334 w344 w355 w373 w382 w390 w418 w426 w433 w443 w446 w450 w463 w472 w481 w491 w500 w507 w513 w516 w520 w524 w533 w542 w552 w563 w565 w568 w578 w580 w586 w588 w590 w593 w596 w598 w600 w612 w624 w635 w638 w640 w655 w658 w663 w677 w690 w692 w697 w699 w700 w702 w704 w707 w709 w723 w740 w769 w780 w792 w796 w797 w802 w808 w813 w816 w827] -> w267
              tunnel: w264 -> [_ w279 _ _ w301 _ _ w317 _ w343 w353 w371 w380 _ w416 _ w432 _ _ w449 w461 w470 w479 w489 w499 w506 _ _ _ _ _ w540 _ _ _ w566 _ _ _ _ _ _ _ _ _ _ _ _ _ _ _ _ _ _ _ _ _ _ _ _ _ _ _ w722 _ _ w779 _ _ _ w801 _ _ w819 _]
              event "Move target", "Slide": Value Change {
                n163 = event-data() -> ("NewVal"=w271:variant)  [unwired: 1 in, 5 out]
                n164 = stacked-sequence {
                  tunnel: w271 -> [_ w278]
                  frame #0 {
                    n165 = local write "cellule"("Slide") -> ()
                    n166 = property on="Cell in place" class="Bool (strict)"("Value"=FALSE ("Cell in place")) -> ()  [unwired: 2 in, 2 out]
                  }
                  frame #1 {
                    n167 = control-ref of="Cell in place"() -> (w277:refnum<vi>)
                    n168 = call "move-targer-eventSD.vi"("cellule"="cellule", "NewVal"=w278, "reference in"=w277, "pos of targets"="pos of targets") -> ()
                  }
                }
              }
              event "STOP": Value Change {
                n169 = event-data() -> ()  [unwired: 1 in, 6 out]
                n170 = flat-sequence {
                  tunnel: [w285] -> w281
                  tunnel: w279 -> [w283]
                  frame #0 {
                    n171 = Unbundle By Name(w283) -> ("Stop event"=w282:refnum<user-event>)
                    n172 = call "stop-eventSD.vi"("Stop Event in"=w282) -> (1:"Cell in place"=w285:bool, 2:"Cell in place"=→"Cell in place":bool)
                  }
                }
              }
              event "Move delay line": Value Change {
                n173 = event-data() -> ("NewVal"=w286:bool)  [unwired: 1 in, 5 out]
                n174 = case shown="Vrai" w286 {
                  frame False {
                  }
                  frame True {
                    n175 = control-ref of="deplacement boolean"() -> (w293:refnum<vi>)
                    n176 = call "move-delayline-eventSD.vi"("Delay pos (mm)"="Delay (mm) 2", "choix cible"="type of movement", "deplacement in"=w293) -> ("Delay (ps)"=→"Delay (ps)":dbl, "moved"=→"moved":string, "Delay (mm)"=→"Delay (mm)":dbl, "deplacement boolean"=→"deplacement boolean":bool)
                  }
                }
              }
              event "Upload wavelength": Value Change {
                n177 = event-data() -> ("NewVal"=w296:bool)  [unwired: 1 in, 5 out]
                n178 = stacked-sequence {
                  tunnel: w296 -> [_ _]
                  frame #0 {
                    n179 = local read "Adress wavelength array"() -> (w298:path)
                    n180 = call "Open_abscisseSD.vi"("wavelengts path"=w298) -> ("wavelengths"=w297:dbl[])
                    n181 = global write "globalVarSD.vi" "wavelengths"(w297) -> ()
                    n182 = local write "wavelengths"(w297) -> ()
                  }
                  frame #1 {
                    n183 = call "verify-selected-wavesSD.vi"("selected wavelengths"="sel. wavelen.") -> ("selected wavelengths out"=w299:dbl[])  [unwired: 1 in, 3 out]
                    n184 = local write "sel. wavelen."(w299) -> ()
                  }
                }
              }
              event "Real time": Value Change {
                n185 = event-data() -> ("NewVal"=w303:bool)  [unwired: 1 in, 5 out]
                n186 = stacked-sequence {
                  tunnel: w303 -> [w306 w309]
                  tunnel: w301 -> [w305 w308]
                  frame #0 {
                    # "Notifies reglage event"
                    n187 = Unbundle By Name(w305) -> ("notifier reglage out"=w304:refnum<notifier>)
                    n188 = Send Notification(notification=w306, notifier=w304) -> ()  [unwired: 1 in, 2 out]
                  }
                  frame #1 {
                    # "Generate reglage event\nwhich activates event in parrallel loop"
                    n189 = Unbundle By Name(w308) -> ("Reglage event"=w307:refnum<user-event>)
                    n190 = case shown="Vrai" w309 {
                      tunnel: w307 -> [_ w310]
                      frame False {
                      }
                      frame True {
                        n191 = Generate User Event(user event=w310, event data cluster=cluster{"Operate":bool} {"Operate"=TRUE} ("event data")) -> ()  [unwired: 2 in, 2 out]
                      }
                    }
                  }
                }
              }
              event "# par point": Value Change {
                n192 = event-data() -> ("NewVal"=w313:i32)  [unwired: 1 in, 5 out]
                n193 = global write "globalVarSD.vi" "Nombre d'acquisition par point (réglage)"(w313) -> ()
              }
              event "# par point": Value Change {
                n194 = event-data() -> ("NewVal"=w314:i32)  [unwired: 1 in, 5 out]
                n195 = flat-sequence {
                  tunnel: w314 -> [w316]
                  frame #0 {
                    n196 = property on="slider" class="Gliss (strict)"("Scale.Maximum"=w316) -> ()  [unwired: 2 in, 2 out]
                    n197 = global write "globalVarSD.vi" "# d'acquisition par point"(w316) -> ()
                  }
                }
              }
              event "Start measurement": Value Change {
                n198 = event-data() -> ("NewVal"=w320:bool)  [unwired: 1 in, 5 out]
                n199 = stacked-sequence {
                  tunnel: w320 -> [_ w332]
                  tunnel: [_ w330] -> w319
                  tunnel: w318 -> [_ w329]
                  tunnel: w317 -> [_ w325]
                  frame #0 {
                    n200 = property on="slider" class="Gliss (strict)"("Scale.Maximum"="# par point") -> ()  [unwired: 2 in, 2 out]
                    n201 = global write "globalVarSD.vi" "# d'acquisition par point"("# par point") -> ()
                    n202 = global write "globalVarSD.vi" "error min"("error min") -> ()
                  }
                  frame #1 {
                    n203 = Unbundle By Name(w325) -> ("notifier mesure out"=w324:refnum<notifier>, "Measure event"=w323:refnum<user-event>)
                    n204 = control-ref of="# current"() -> (w331:refnum<vi>)
                    n205 = global write "globalVarSD.vi" "# points"("# points") -> ()
                    n206 = call "start-measurement-eventSD.vi"("# current"=w331, "NewVal"=w332, "cluster in"=w329, "Measure event"=w323, "notifier mesure in"=w324) -> ("cluster out"=w330:T13)
                    n207 = global write "globalVarSD.vi" "delay0"("OZ, ps") -> ()
                    n208 = global write "globalVarSD.vi" "deltaT"("step, ps") -> ()
                  }
                }
              }
              event "add group": Value Change {
                n209 = event-data() -> ("NewVal"=w333:bool)  [unwired: 1 in, 5 out]
                n210 = case shown="Vrai" w333 {
                  tunnel: w335 -> [w336 w342]
                  tunnel: [w336 w341] -> w334
                  frame False {
                  }
                  frame True {
                    n211 = local read "save Radio Buttons"() -> (w340:enum32{"Automatic", "User-def"})
                    n212 = control-ref of="group"() -> (w337:refnum<vi>)
                    n213 = call "add-group-eventSD.vi"("Commentaires group"="Commentaires group", "cluster in"=w342, "save Radio Buttons"=w340, "Name group"="Name group", "Group"=w337) -> ("cluster out"=w341:T13)
                  }
                }
              }
              event "group": Value Change {
                n214 = event-data() -> ("NewVal"=w346:u16)  [unwired: 1 in, 5 out]
                n215 = flat-sequence {
                  tunnel: w346 -> [w352]
                  tunnel: w345 -> [w351]
                  tunnel: [w350] -> w344
                  tunnel: w343 -> [w348]
                  frame #0 {
                    n216 = Unbundle By Name(w348) -> ("Update graphs of exp"=w347:refnum<user-event>)
                    n217 = call "group-change-eventSD.vi"("cluster in"=w351, "group new value"=w352, "User Event in"=w347) -> ("String"=w349:string, "cluster out"=w350:T13)
                    n218 = local write "Commentaires group"(w349) -> ()
                  }
                }
              }
              event "add exp": Value Change {
                n219 = event-data() -> ("NewVal"=w354:bool)  [unwired: 1 in, 5 out]
                n220 = case shown="Vrai" w354 {
                  tunnel: w356 -> [w357 w370]
                  tunnel: [w357 w369] -> w355
                  tunnel: w353 -> [_ w359]
                  frame False {
                  }
                  frame True {
                    n221 = Unbundle By Name(w359) -> ("Update graphs of exp"=w358:refnum<user-event>)
                    n222 = local read "step, ps"() -> (w362:dbl)
                    n223 = local read "OZ, ps"() -> (w361:dbl)
                    n224 = local read "# points"() -> (w363:i32)
                    n225 = Bundle By Name(cluster=T9 {"Fix"=TRUE, "DeltaT"=0.0, "#points"=0, "Delay"=0.0}, "Fix"="Fix", "DeltaT"=w362, "#points"=w363, "Delay"=w361) -> (w360:T9)
                    n226 = call "add-exp-eventSD.vi"("Exp name"="Exp name", "Update graphs of exp"=w358, "add exp"="add exp", "cluster in"=w370, "Commentaires exp"="Commentaires exp", "Bounds"=w360) -> ("cluster out"=w369:T13)  [unwired: 1 in]
                  }
                }
              }
              event Double Click {
                n227 = event-data() -> ("Row"=w374:i32)  [unwired: 1 in, 8 out]
                n228 = flat-sequence {
                  tunnel: w374 -> [w379]
                  tunnel: w372 -> [w378]
                  tunnel: [w377] -> w373
                  tunnel: w371 -> [w376]
                  frame #0 {
                    n229 = Unbundle By Name(w376) -> ("Update graphs of exp"=w375:refnum<user-event>)
                    n230 = call "exp-doubleclick-eventSD.vi"("cluster in"=w378, "Row"=w379, "Update graphs of exp"=w375) -> ("cluster out"=w377:T13)
                  }
                }
              }
              event "del group": Value Change {
                n231 = event-data() -> ("NewVal"=w381:bool)  [unwired: 1 in, 5 out]
                n232 = case shown="Vrai" w381 {
                  tunnel: w383 -> [w384 w389]
                  tunnel: [w384 w388] -> w382
                  tunnel: w380 -> [_ w386]
                  frame False {
                  }
                  frame True {
                    n233 = Unbundle By Name(w386) -> ("Update graphs of exp"=w385:refnum<user-event>)
                    n234 = call "del-group-eventSD.vi"("cluster in"=w389, "User Event in"=w385) -> ("cluster out"=w388:T13)
                    n235 = Unbundle By Name(w388) -> ("group"=w387:i32)
                    n236 = local write "group"(w387) -> ()
                  }
                }
              }
              event User Event {
                n237 = event-data() -> ("Full/Part"=w394:bool, "Item names"=w393:string[], "Exp number"=w392:i32)  [unwired: 1 in, 4 out]
                n238 = stacked-sequence {
                  seq-local: [w395 _] -> [_ w415]
                  tunnel: w394 -> [w404 _]
                  tunnel: w393 -> [w403 _]
                  tunnel: w392 -> [w402 _]
                  tunnel: w391 -> [w396 _]
                  tunnel: [_ w413] -> w390
                  frame #0 {
                    n239 = local read "mimic main cursor move"() -> (w400:bool)
                    n240 = control-ref of="Commentaires exp"() -> (w397:refnum<vi>)
                    n241 = control-ref of="group"() -> (w399:refnum<vi>)
                    n242 = control-ref of="group"() -> (w398:refnum<vi>)
                    n243 = call "update-grapheventSD.vi"("Exp number"=w402, "Full/Part"=w404, "Item names"=w403, "mimic cursor move"=w400, "cluster in"=w396, "Commentaires exp"=w397, "group"=w398, "Ring in"=w399) -> ("cluster out"=w395:T13, "Boolean"=w401:bool)
                    n244 = property on="mimic main cursor move" class="Bool (strict)"("Val(Sgnl)"=w401) -> ()  [unwired: 2 in, 2 out]
                  }
                  frame #1 {
                    n245 = call "update_param_expSD.vi"("cluster in"=w415) -> ("numberpoints, ps"=w405:i32, "deltaTlast"=w406:dbl, "# current"=w408:i32, "Delay0,ps"=w407:dbl, "cluster out"=w414:T13)  [unwired: 4 in, 1 out]
                    n246 = local write "# current"(w408) -> ()
                    n247 = call "calc-total-kinetics.vi"("cluster in"=w414, "delay0"=w407, "# points"=w405, "deltaT"=w406) -> ("cluster out"=w413:T13, "Real delay time, ps"=→"RDT, ps":dbl, "Kinetics, ps"=w411:dbl, "Total, ps"=w412:dbl, "# points out"=w409:i32)  [unwired: 1 in]
                    n248 = local write "# points"(w409) -> ()
                    n249 = local write "step, ps"(w406) -> ()
                    n250 = local write "OZ, ps"(w407) -> ()
                    n251 = local write "Total, ps"(w412) -> ()
                    n252 = local write "Kinetics, ps"(w411) -> ()
                  }
                }
              }
              event "del exp": Value Change {
                n253 = event-data() -> ("NewVal"=w417:bool)  [unwired: 1 in, 5 out]
                n254 = case shown="Vrai" w417 {
                  tunnel: w419 -> [w420 w424]
                  tunnel: [w420 w423] -> w418
                  tunnel: w416 -> [_ w422]
                  frame False {
                  }
                  frame True {
                    n255 = Unbundle By Name(w422) -> ("Update graphs of exp"=w421:refnum<user-event>)
                    n256 = call "del-exp-eventSD.vi"("cluster in"=w424, "Update graphs of exp"=w421) -> ("cluster out"=w423:T13)
                  }
                }
              }
              event "Save": Value Change {
                n257 = event-data() -> ("NewVal"=w425:bool)  [unwired: 1 in, 5 out]
                n258 = case shown="Vrai" w425 {
                  tunnel: w427 -> [w428 w431]
                  tunnel: [w428 w430] -> w426
                  frame False {
                  }
                  frame True {
                    n259 = call "save-eventSD.vi"("cluster in"=w431, "save Radio Buttons"="save Radio Buttons") -> ("cluster out"=w430:T13)
                  }
                }
              }
              event User Event {
                n260 = event-data() -> ("Experiment"=w435:refnum<class "Experiment.lvclass">)  [unwired: 1 in, 5 out]
                n261 = stacked-sequence {
                  tunnel: w435 -> [w440 _]
                  tunnel: w434 -> [w439 _]
                  tunnel: [w438 _] -> w433
                  tunnel: w432 -> [w437 _]
                  frame #0 {
                    n262 = Unbundle By Name(w437) -> ("Update graphs of exp"=w436:refnum<user-event>)
                    n263 = call "measurement-finished-eventSD.vi"("cluster in"=w439, "Update graphs of exp"=w436, "Experiment in"=w440) -> ("cluster out"=w438:T13)
                  }
                  frame #1 {
                    n264 = local read "mimic main cursor move"() -> (w442:bool)
                    n265 = Not(x=w442) -> (.not. x?=w441:bool)
                    n266 = property on="mimic main cursor move" class="Bool (strict)"("Val(Sgnl)"=w441) -> ()  [unwired: 2 in, 2 out]
                  }
                }
              }
              event "Commentaires group": Value Change {
                n267 = event-data() -> ("NewVal"=w445:string)  [unwired: 1 in, 5 out]
                n268 = call "comments-change-group-eventSD.vi"("cluster in"=w444, "NewVal"=w445) -> ("cluster out"=w443:T13)
              }
              event "Commentaires exp": Value Change {
                n269 = event-data() -> ("NewVal"=w448:string)  [unwired: 1 in, 5 out]
                n270 = call "comments-change-eventSD.vi"("cluster in"=w447, "NewVal"=w448) -> ("cluster out"=w446:T13)
              }
              event "GRAPH EXPERIMENTAL DATA": Cursor Move; "mimic main cursor move": Value Change {
                n271 = event-data() -> ()  [unwired: 1 in, 4 out]
                n272 = stacked-sequence {
                  tunnel: w451 -> [_ w460]
                  tunnel: [_ w459] -> w450
                  tunnel: w449 -> [_ w453]
                  frame #0 {
                    n273 = local write "Block"(FALSE) -> ()
                  }
                  frame #1 {
                    n274 = Unbundle By Name(w453) -> ("redraw event"=w454:refnum<user-event>)
                    n275 = call "cursor-moveSD.vi"("cluster in"=w460, "User Event in"=w454) -> ("output out"=w459:T13)
                    n276 = Unbundle By Name(w459) -> ("FromToWave.FromWave"=w457:dbl, "FromToWave.ToWave"=w458:dbl, "FromToDelay.FromDelay"=w455:dbl, "FromToDelay.ToDelay"=w456:dbl)
                    n277 = local write "From Time"(w455) -> ()
                    n278 = local write "From Wave"(w457) -> ()
                    n279 = local write "To Wave"(w458) -> ()
                    n280 = local write "To Time"(w456) -> ()
                  }
                }
              }
              event "Add kinetics": Value Change {
                n281 = event-data() -> ("NewVal"=w462:bool)  [unwired: 1 in, 5 out]
                n282 = case shown="Vrai" w462 {
                  tunnel: w464 -> [w465 w469]
                  tunnel: [w465 w468] -> w463
                  tunnel: w461 -> [_ w467]
                  frame False {
                  }
                  frame True {
                    n283 = Unbundle By Name(w467) -> ("redraw event"=w466:refnum<user-event>)
                    n284 = call "add-kintecis-eventSD.vi"("cluster in"=w469, "redraw event"=w466) -> ("cluster out"=w468:T13)
                  }
                }
              }
              event "Add spectrum": Value Change {
                n285 = event-data() -> ("NewVal"=w471:bool)  [unwired: 1 in, 5 out]
                n286 = case shown="Vrai" w471 {
                  tunnel: w473 -> [w474 w478]
                  tunnel: [w474 w477] -> w472
                  tunnel: w470 -> [_ w475]
                  frame False {
                  }
                  frame True {
                    n287 = Unbundle By Name(w475) -> ("redraw event"=w476:refnum<user-event>)
                    n288 = call "add-spectrum-eventSD.vi"("cluster in"=w478, "redraw event"=w476) -> ("cluster out"=w477:T13)
                  }
                }
              }
              event "Del kinetics": Value Change {
                n289 = event-data() -> ("NewVal"=w480:bool)  [unwired: 1 in, 5 out]
                n290 = case shown="Vrai" w480 {
                  tunnel: w482 -> [w483 w488]
                  tunnel: [w483 w487] -> w481
                  tunnel: w479 -> [_ w485]
                  frame False {
                  }
                  frame True {
                    n291 = Unbundle By Name(w485) -> ("redraw event"=w484:refnum<user-event>)
                    n292 = local read "sel kin"() -> (w486:i32)
                    n293 = call "del-kinetics-eventSD.vi"("cluster in"=w488, "selected kinetics"=w486, "User Event in"=w484) -> ("cluster out"=w487:T13)
                  }
                }
              }
              event "Del spectrum": Value Change {
                n294 = event-data() -> ("NewVal"=w490:bool)  [unwired: 1 in, 5 out]
                n295 = case shown="Vrai" w490 {
                  tunnel: w492 -> [w493 w498]
                  tunnel: [w493 w497] -> w491
                  tunnel: w489 -> [_ w494]
                  frame False {
                  }
                  frame True {
                    n296 = Unbundle By Name(w494) -> ("redraw event"=w495:refnum<user-event>)
                    n297 = local read "sel spect"() -> (w496:i32)
                    n298 = call "del-spectrum-eventSD.vi"("cluster in"=w498, "selected spectrum"=w496, "User Event in"=w495) -> ("cluster out"=w497:T13)
                  }
                }
              }
              event "Avr kinetics": Value Change {
                n299 = event-data() -> ()  [unwired: 1 in, 6 out]
                n300 = flat-sequence {
                  tunnel: w501 -> [w505]
                  tunnel: [w504] -> w500
                  tunnel: w499 -> [w503]
                  frame #0 {
                    n301 = Unbundle By Name(w503) -> ("redraw event"=w502:refnum<user-event>)
                    n302 = call "average-kin-eventSD.vi"("User Event in"=w502, "cluster in"=w505) -> ("cluster out"=w504:T13)
                  }
                }
              }
              event "Avr spectrum": Value Change {
                n303 = event-data() -> ()  [unwired: 1 in, 6 out]
                n304 = flat-sequence {
                  tunnel: w508 -> [w512]
                  tunnel: [w511] -> w507
                  tunnel: w506 -> [w509]
                  frame #0 {
                    n305 = Unbundle By Name(w509) -> ("redraw event"=w510:refnum<user-event>)
                    n306 = call "average-spectra-eventSD.vi"("User Event in"=w510, "cluster in"=w512) -> ("cluster out"=w511:T13)
                  }
                }
              }
              event "Spectrum O.D.": Shortcut Menu Selection (User) {
                n307 = event-data() -> ("ItemTag"=w515:string)  [unwired: 1 in, 7 out]
                n308 = call "copy-spectrum-eventSD.vi"("cluster in"=w514, "ItemTag"=w515) -> ("cluster out"=w513:T13)
              }
              event "Kinetics": Shortcut Menu Selection (User) {
                n309 = event-data() -> ("ItemTag"=w518:string)  [unwired: 1 in, 7 out]
                n310 = call "copy-kinetics-eventSD.vi"("cluster in"=w517, "ItemTag"=w518) -> ("cluster out"=w516:T13)
              }
              event "GRAPH EXPERIMENTAL DATA": Shortcut Menu Selection (User) {
                n311 = event-data() -> ("ItemTag"=w522:string)  [unwired: 1 in, 7 out]
                n312 = local read "sel. wavelen."() -> (w519:dbl[])
                n313 = call "copy-data-eventSD.vi"("cluster in"=w521, "selected wavelengths"=w519, "ItemTag"=w522) -> ("cluster out"=w520:T13)
              }
              event "def pixel+", "def pixel-": Value Change {
                n314 = event-data() -> ("NewVal"=w525:dbl)  [unwired: 1 in, 5 out]
                n315 = flat-sequence {
                  tunnel: w525 -> [w532]
                  tunnel: [w527] -> w524
                  tunnel: w523 -> [w526]
                  frame #0 {
                    n316 = call "BG-change-pixel-eventSD.vi"("def pixel lower"="def pixel-", "def pixel upper"="def pixel+", "NewVal"=w532, "cluster in"=w526, "mimic cursor move"="mimic main cursor move") -> ("Boolean"=w529:bool, "cluster out"=w527:T13)
                    n317 = property on="mimic main cursor move" class="Bool (strict)"("Val(Sgnl)"=w529) -> ()  [unwired: 2 in, 2 out]
                  }
                }
              }
              event "Kinetics": Cursor Move {
                n318 = event-data() -> ()  [unwired: 1 in, 4 out]
                n319 = flat-sequence {
                  tunnel: w534 -> [w539]
                  tunnel: [w538] -> w533
                  frame #0 {
                    n320 = control-ref of="Kinetics"() -> (w537:refnum<vi>)
                    n321 = property on="mimic main cursor move" class="Bool (strict)"() -> ("Value"=w536:bool)  [unwired: 2 in, 2 out]
                    n322 = call "clean-change-cursor-kin-event.vi"("cluster in"=w539, "Kinetics graph"=w537) -> ("cluster out"=w538:T13)
                    n323 = Not(x=w536) -> (.not. x?=w535:bool)
                    n324 = property on="mimic main cursor move" class="Bool (strict)"("Val(Sgnl)"=w535) -> ()  [unwired: 2 in, 2 out]
                  }
                }
              }
              event "BG correct": Value Change {
                n325 = event-data() -> ("NewVal"=w541:bool)  [unwired: 1 in, 5 out]
                n326 = case shown="Vrai" w541 {
                  tunnel: w543 -> [w544 w551]
                  tunnel: [w544 w550] -> w542
                  tunnel: w540 -> [_ w546]
                  frame False {
                  }
                  frame True {
                    n327 = Unbundle By Name(w546) -> ("Update graphs of exp"=w545:refnum<user-event>)
                    n328 = local read "def pixel+"() -> (w548:dbl)
                    n329 = local read "def pixel-"() -> (w549:dbl)
                    n330 = call "BG-corr-eventSD.vi"("Single"="All", "cluster in"=w551, "Update graphs of exp"=w545, "def pixel lower"=w549, "def pixel upper"=w548) -> ("cluster out"=w550:T13)
                  }
                }
              }
              event User Event {
                n331 = event-data() -> ()  [unwired: 1 in, 5 out]
                n332 = stacked-sequence {
                  tunnel: w552 -> [w553 w559]
                  frame #0 {
                    n333 = Unbundle By Name(w553) -> ("GRAPH EXPERIMENTAL DATA"=→"GRAPH EXPERIMENTAL DATA":dbl[][], "Kinetics"=→"Kinetics":cluster{"timedelay":dbl[], dbl[]}[], "Spectrum"=→"Spectrum O.D.":cluster{"Unités abscisse":dbl[], dbl[]}[])  [unwired: 2 out]
                  }
                  frame #1 {
                    n334 = Unbundle By Name(w559) -> ("kinetics plot names"=w558:string[], "spectra plot names"=w557:string[])
                    n335 = control-ref of="Spectrum O.D."() -> (w561:refnum<vi>)
                    n336 = control-ref of="Kinetics"() -> (w560:refnum<vi>)
                    n337 = call "update-graphlegendOD.vi"("XYGraph in"=w560, "plot names"=w558) -> ()
                    n338 = call "update-graphlegendOD.vi"("XYGraph in"=w561, "plot names"=w557) -> ()
                  }
                }
              }
              event "Spectrum O.D.": Plot Attribute Change {
                n339 = event-data() -> ("PlotIdx"=w562:i32)  [unwired: 1 in, 6 out]
                n340 = property on="sel spect" class="NumNb (strict)"("Value"=w562) -> ()  [unwired: 2 in, 2 out]
                n341 = property on="Spectrum O.D." class="GraphXY (strict)"("Active Plot"=w562) -> ()  [unwired: 2 in, 2 out]
              }
              event "Kinetics": Plot Attribute Change {
                n342 = event-data() -> ("PlotIdx"=w564:i32)  [unwired: 1 in, 7 out]
                n343 = property on="sel kin" class="NumNb (strict)"("Value"=w564) -> ()  [unwired: 2 in, 2 out]
                n344 = property on="Kinetics" class="GraphXY (strict)"("Active Plot"=w564) -> ()  [unwired: 2 in, 2 out]
              }
              event "Average exp": Value Change {
                n345 = event-data() -> ("NewVal"=w567:bool)  [unwired: 1 in, 5 out]
                n346 = case shown="Vrai" w567 {
                  tunnel: w569 -> [w570 w577]
                  tunnel: [w570 w576] -> w568
                  tunnel: w566 -> [_ w572]
                  frame False {
                  }
                  frame True {
                    n347 = property on="Commentaires exp" class="Ch"() -> ("Value"=w574:string)  [unwired: 2 in, 2 out]
                    n348 = property on="Exp name" class="Ch"() -> ("Value"=w575:string)  [unwired: 2 in, 2 out]
                    n349 = Unbundle By Name(w572) -> ("Update graphs of exp"=w571:refnum<user-event>)
                    n350 = Bundle("Value"=w575, "Value"=w574) -> (w573:cluster{"Value":string, "Value":string})  [unwired: 1 in]
                    n351 = call "average-exp-eventSD.vi"("cluster in"=w577, "Update graphs of exp"=w571, "Name cluster"=w573) -> ("cluster out"=w576:T13)
                  }
                }
              }
              event "shift": Value Change {
                n352 = event-data() -> ("NewVal"=w579:i32)  [unwired: 1 in, 5 out]
                n353 = global write "globalVarSD.vi" "shift"(w579) -> ()
              }
              event "Save SC": Value Change {
                n354 = event-data() -> ("NewVal"=w582:bool)  [unwired: 1 in, 5 out]
                n355 = case shown="Vrai" w582 {
                  tunnel: w581 -> [w583 w585]
                  tunnel: [w583 w584] -> w580
                  frame False {
                  }
                  frame True {
                    n356 = call "SC-save_eventSD.vi"("cluster in"=w585) -> ("cluster out"=w584:T13)
                  }
                }
              }
              event "error min": Value Change {
                n357 = event-data() -> ("NewVal"=w587:dbl)  [unwired: 1 in, 5 out]
                n358 = global write "globalVarSD.vi" "error min"(w587) -> ()
              }
              event "Log": Value Change {
                n359 = event-data() -> ("NewVal"=w589:bool)  [unwired: 1 in, 5 out]
                n360 = global write "globalVarSD.vi" "Log"(w589) -> ()
              }
              event "sel spect": Value Change {
                n361 = event-data() -> ("NewVal"=w591:i32)  [unwired: 1 in, 5 out]
                n362 = flat-sequence {
                  tunnel: w591 -> [w592]
                  frame #0 {
                    n363 = property on="Spectrum O.D." class="GraphXY (strict)"("Active Plot"=w592) -> ()  [unwired: 2 in, 2 out]
                  }
                }
              }
              event "sel kin": Value Change {
                n364 = event-data() -> ("NewVal"=w594:i32)  [unwired: 1 in, 5 out]
                n365 = flat-sequence {
                  tunnel: w594 -> [w595]
                  frame #0 {
                    n366 = property on="Kinetics" class="GraphXY (strict)"("Active Plot"=w595) -> ()  [unwired: 2 in, 2 out]
                  }
                }
              }
              event "pixel-": Value Change {
                n367 = event-data() -> ("NewVal"=w597:i32)  [unwired: 1 in, 5 out]
                n368 = global write "globalVarSD.vi" "pixel-"(w597) -> ()
              }
              event "pixel+": Value Change {
                n369 = event-data() -> ("NewVal"=w599:i32)  [unwired: 1 in, 5 out]
                n370 = global write "globalVarSD.vi" "pixel+"(w599) -> ()
              }
              event "OZ, ps": Value Change {
                n371 = event-data() -> ("NewVal"=w602:dbl)  [unwired: 1 in, 5 out]
                n372 = flat-sequence {
                  tunnel: w602 -> [w606]
                  tunnel: w601 -> [w604]
                  tunnel: [w603] -> w600
                  frame #0 {
                    n373 = global write "globalVarSD.vi" "delay0"(w606) -> ()
                    n374 = local read "step, ps"() -> (w611:dbl)
                    n375 = local read "# points"() -> (w610:i32)
                    n376 = call "calc-total-kinetics.vi"("cluster in"=w604, "delay0"=w606, "# points"=w610, "deltaT"=w611) -> ("cluster out"=w603:T13, "Real delay time, ps"=w605:dbl, "Kinetics, ps"=w608:dbl, "Total, ps"=→"Total, ps":dbl, "# points out"=w607:i32)  [unwired: 1 in]
                    n377 = local write "# points"(w607) -> ()
                    n378 = global write "globalVarSD.vi" "# points"(w607) -> ()
                    n379 = property on="Kinetics, ps" class="NumNb (strict)"("Value"=w608) -> ()  [unwired: 2 in, 2 out]
                    n380 = local write "RDT, ps"(w605) -> ()
                  }
                }
              }
              event "step, ps": Value Change {
                n381 = event-data() -> ("NewVal"=w614:dbl)  [unwired: 1 in, 5 out]
                n382 = flat-sequence {
                  tunnel: w614 -> [w616]
                  tunnel: w613 -> [w619]
                  tunnel: [w618] -> w612
                  frame #0 {
                    n383 = local read "OZ, ps"() -> (w615:dbl)
                    n384 = global write "globalVarSD.vi" "deltaT"(w616) -> ()
                    n385 = local read "# points"() -> (w623:i32)
                    n386 = call "calc-total-kinetics.vi"("cluster in"=w619, "delay0"=w615, "# points"=w623, "deltaT"=w616) -> ("cluster out"=w618:T13, "Real delay time, ps"=w617:dbl, "Kinetics, ps"=→"Kinetics, ps":dbl, "Total, ps"=w622:dbl, "# points out"=w620:i32)  [unwired: 1 in]
                    n387 = local write "Total, ps"(w622) -> ()
                    n388 = local write "# points"(w620) -> ()
                    n389 = global write "globalVarSD.vi" "# points"(w620) -> ()
                    n390 = local write "RDT, ps"(w617) -> ()
                  }
                }
              }
              event "aq contol": Value Change {
                n391 = event-data() -> ("NewVal"=w625:enum32{"fixed", "automatic", "fixed-auto"})  [unwired: 1 in, 5 out]
                n392 = flat-sequence {
                  tunnel: w625 -> [w628]
                  frame #0 {
                    n393 = case shown="\"fixed-auto\"" w628 {
                      tunnel: [FALSE TRUE FALSE] -> w627
                      tunnel: [FALSE FALSE TRUE] -> w626
                      frame "fixed", Default {
                      }
                      frame "automatic" {
                      }
                      frame "fixed-auto" {
                      }
                    }
                    n394 = property on="Break measurement" class="Bool (strict)"("Visible"=w626) -> ()  [unwired: 2 in, 2 out]
                    n395 = property on="error" class="BoutRot (strict)"("Visible"=w627) -> ()  [unwired: 2 in, 2 out]
                    n396 = property on="slider" class="Gliss (strict)"("Visible"=w627) -> ()  [unwired: 2 in, 2 out]
                    n397 = property on="error min" class="NumNb (strict)"("Visible"=w627) -> ()  [unwired: 2 in, 2 out]
                  }
                }
              }
              event "Statistics": Value Change {
                n398 = event-data() -> ("NewVal"=w636:bool)  [unwired: 1 in, 5 out]
                n399 = case shown="Vrai" w636 {
                  frame False {
                  }
                  frame True {
                    n400 = call "statistics-deviation.vi"() -> ()  [unwired: 12 in]
                  }
                }
              }
              event "Old/New": Value Change {
                n401 = event-data() -> ("NewVal"=w637:bool)  [unwired: 1 in, 5 out]
                n402 = global write "globalVarSD.vi" "Old/New"(w637) -> ()
              }
              event "cooling": Value Change {
                n403 = event-data() -> ("NewVal"=w641:bool)  [unwired: 1 in, 5 out]
                n404 = flat-sequence {
                  tunnel: w641 -> [w647]
                  tunnel: w639 -> [w644]
                  tunnel: [w645] -> w640
                  frame #0 {
                    n405 = Unbundle By Name(w644) -> ("error out"=w643:errorcluster)
                    n406 = Not(x=w647) -> (.not. x?=w642:bool)
                    n407 = case shown="Vrai" w642 {
                      tunnel: [w649 w652] -> w646
                      tunnel: w643 -> [w648 w651]
                      frame False {
                        n408 = call "CoolerOFFSD.vi"("error in (no error)"=w648) -> ("error out"=w649:errorcluster)  [unwired: 1 in, 1 out]
                      }
                      frame True {
                        n409 = control-ref of="Thermometer"() -> (w650:refnum<vi>)
                        n410 = call "Cooldetector-uv-visSD.vi"("error in (no error)"=w651, "Thermometer"=w650, "temp set"="temp set") -> ("error out"=w652:errorcluster, "status"=→"status cooling process":T6)
                      }
                    }
                    n411 = Bundle By Name(cluster=w644, "error out"=w646) -> (w645:T13)
                  }
                }
              }
              event "Check T": Value Change {
                n412 = event-data() -> ("NewVal"=w656:bool)  [unwired: 1 in, 5 out]
                n413 = case shown="Vrai" w656 {
                  frame False {
                  }
                  frame True {
                    n414 = call "GetTemperatureSD.vi"() -> ("temperature"=→"Thermometer":i32)  [unwired: 4 in, 3 out]
                  }
                }
              }
              event "load table": Value Change {
                n415 = event-data() -> ("NewVal"=w659:bool)  [unwired: 1 in, 5 out]
                n416 = case shown="Vrai" w659 {
                  frame False {
                  }
                  frame True {
                    n417 = local read "Table path"() -> (w661:path)
                    n418 = call "Open_abscisseSD.vi"("wavelengts path"=w661) -> ("wavelengths"=w660:dbl[])
                    n419 = local write "table delays"(w660) -> ()
                  }
                }
              }
              event "From Wave", "To Wave": Value Change {
                n420 = event-data() -> ()  [unwired: 1 in, 6 out]
                n421 = local read "Block"() -> (w662:bool)
                n422 = case shown="Faux" w662 {
                  selector: w662 -> [w665 w674]
                  tunnel: w664 -> [w667 w675]
                  tunnel: [w666 w675] -> w663
                  frame False {
                    n423 = stacked-sequence {
                      tunnel: w667 -> [w671 _]
                      tunnel: [w670 _] -> w666
                      tunnel: w665 -> [_ w672]
                      frame #0 {
                        n424 = local read "From Wave"() -> (w669:dbl)
                        n425 = local read "To Wave"() -> (w668:dbl)
                        n426 = call "change-waveposSD.vi"("ToWave"=w668, "FromWave"=w669, "cluster in"=w671) -> ("cluster in out"=w670:T13)
                      }
                      frame #1 {
                        n427 = property on="mimic main cursor move" class="Bool (strict)"("Val(Sgnl)"=w672) -> ()  [unwired: 2 in, 2 out]
                      }
                    }
                  }
                  frame True {
                    n428 = Not(x=w674) -> (.not. x?=w673:bool)
                    n429 = local write "Block"(w673) -> ()
                  }
                }
              }
              event "From Time", "To Time": Value Change {
                n430 = event-data() -> ()  [unwired: 1 in, 6 out]
                n431 = local read "Block"() -> (w676:bool)
                n432 = case shown="Faux" w676 {
                  selector: w676 -> [w679 w688]
                  tunnel: w678 -> [w681 w689]
                  tunnel: [w680 w689] -> w677
                  frame False {
                    n433 = stacked-sequence {
                      tunnel: w681 -> [w685 _]
                      tunnel: [w684 _] -> w680
                      tunnel: w679 -> [_ w686]
                      frame #0 {
                        n434 = local read "From Time"() -> (w683:dbl)
                        n435 = local read "To Time"() -> (w682:dbl)
                        n436 = call "change-timeposSD.vi"("ToTime"=w682, "FromTime"=w683, "cluster in"=w685) -> ("cluster in out"=w684:T13)
                      }
                      frame #1 {
                        n437 = property on="mimic main cursor move" class="Bool (strict)"("Val(Sgnl)"=w686) -> ()  [unwired: 2 in, 2 out]
                      }
                    }
                  }
                  frame True {
                    n438 = Not(x=w688) -> (.not. x?=w687:bool)
                    n439 = local write "Block"(w687) -> ()
                  }
                }
              }
              event "Base path": Value Change {
                n440 = event-data() -> ("NewVal"=w691:path)  [unwired: 1 in, 5 out]
                n441 = global write "globalVarSD.vi" "BasePath"(w691) -> ()
              }
              event "sel. wavelen.": Value Change {
                n442 = event-data() -> ("NewVal"=w693:dbl[])  [unwired: 1 in, 5 out]
                n443 = flat-sequence {
                  tunnel: w693 -> [w694]
                  frame #0 {
                    n444 = call "verify-selected-wavesSD.vi"("selected wavelengths"=w694) -> ("selected wavelengths out"=w695:dbl[])  [unwired: 1 in, 3 out]
                    n445 = local write "sel. wavelen."(w695) -> ()
                  }
                }
              }
              event "Pixel test": Value Change {
                n446 = event-data() -> ("NewVal"=w696:i32)  [unwired: 1 in, 5 out]
                n447 = global write "globalVarSD.vi" "Pixel test"(w696) -> ()
              }
              event "Seuil SC Ref": Value Change {
                n448 = event-data() -> ("NewVal"=w698:dbl)  [unwired: 1 in, 5 out]
                n449 = global write "globalVarSD.vi" "Seuil SC Ref"(w698) -> ()
              }
              event "Seuil SC Sig": Value Change {
                n450 = event-data() -> ("NewVal"=w701:dbl)  [unwired: 1 in, 5 out]
                n451 = global write "globalVarSD.vi" "Seuil SC Sig"(w701) -> ()
              }
              event "Cut On/off": Value Change {
                n452 = event-data() -> ("NewVal"=w703:bool)  [unwired: 1 in, 5 out]
                n453 = global write "globalVarSD.vi" "Cut ON/OFF"(w703) -> ()
              }
              event "real Zero": Value Change {
                n454 = event-data() -> ("NewVal"=w705:dbl)  [unwired: 1 in, 5 out]
                n455 = global write "globalVarSD.vi" "Real zero"(w705) -> ()
              }
              event Edit Cell {
                n456 = event-data() -> ("String"=w706:string)  [unwired: 1 in, 5 out]
                n457 = call "exp-list-nameeditSD.vi"("cluster in"=w708, "new name"=w706) -> ("cluster out"=w707:T13)
              }
              event "# points": Value Change {
                n458 = event-data() -> ("NewVal"=w711:i32)  [unwired: 1 in, 5 out]
                n459 = stacked-sequence {
                  tunnel: w711 -> [w721]
                  tunnel: w710 -> [w714]
                  tunnel: [w713] -> w709
                  frame #0 {
                    n460 = global write "globalVarSD.vi" "# points"(w721) -> ()
                    n461 = local read "step, ps"() -> (w718:dbl)
                    n462 = local read "OZ, ps"() -> (w716:dbl)
                    n463 = local read "# points"() -> (w719:i32)
                    n464 = call "calc-total-kinetics.vi"("cluster in"=w714, "delay0"=w716, "# points"=w719, "deltaT"=w718) -> ("cluster out"=w713:T13, "Real delay time, ps"=w712:dbl, "Kinetics, ps"=w717:dbl, "Total, ps"=w720:dbl, "# points out"=w715:i32)  [unwired: 1 in]
                    n465 = property on="Kinetics, ps" class="NumNb (strict)"("Value"=w717) -> ()  [unwired: 2 in, 2 out]
                    n466 = global write "globalVarSD.vi" "# points"(w715) -> ()
                    n467 = local write "# points"(w715) -> ()
                    n468 = local write "Total, ps"(w720) -> ()
                    n469 = local write "RDT, ps"(w712) -> ()
                  }
                }
              }
              event "load Exp": Value Change {
                n470 = event-data() -> ("NewVal"=w725:bool)  [unwired: 1 in, 5 out]
                n471 = case shown="Vrai" w725 {
                  tunnel: w724 -> [w726 w733]
                  tunnel: [w726 w736] -> w723
                  tunnel: w722 -> [_ w728]
                  frame False {
                  }
                  frame True {
                    n472 = Unbundle By Name(w733) -> ("Experiments groups"=w732:refnum<class "Experiments_group.lvclass">[], "group"=w731:i32)
                    n473 = control-ref of="group"() -> (w734:refnum<vi>)
                    n474 = Index Array(array=w732, index=w731) -> (element=w730:refnum<class "Experiments_group.lvclass">)
                    n475 = call-dynamic "get_path_group.vi"("Experiments_group.lvclass in"=w730) -> ("Path"=w729:path)  [unwired: 1 in, 2 out]
                    n476 = call "Multi-Selection-Dialog-Box.vi"("Start In"=w729, "Group"=w734, "cluster in"=w733) -> ("String File Names"=w737:string[], "cluster out"=w736:T13)  [unwired: 1 out]
                    n477 = Unbundle By Name(w728) -> ("Update graphs of exp"=w727:refnum<user-event>)
                    n478 = Unbundle By Name(w736) -> ("exp selected"=w735:i32)
                    n479 = Bundle(FALSE, "String File Names"=w737, "exp selected"=w735) -> (w738:T16)  [unwired: 1 in]
                    n480 = Generate User Event(user event=w727, event data cluster=w738) -> ()  [unwired: 2 in, 2 out]
                  }
                }
              }
              event "Move Crystall": Value Change {
                n481 = event-data() -> ("NewVal"=w742:bool)  [unwired: 1 in, 5 out]
                n482 = case shown="Vrai" w742 {
                  tunnel: w741 -> [w743 w746]
                  tunnel: [w743 w745] -> w740
                  frame False {
                  }
                  frame True {
                    n483 = Unbundle By Name(w746) -> ("Motor task"=w748:refnum<k21>, "error out"=w747:errorcluster)
                    n484 = flat-sequence {
                      tunnel: "Time, ms" -> [w756]
                      tunnel: [w759] -> w753
                      tunnel: [w758] -> w751
                      tunnel: w748 -> [w757]
                      tunnel: [w756] -> w749
                      tunnel: w747 -> [w755]
                      tunnel: w753 -> [w763]
                      tunnel: [w763] -> w752
                      tunnel: w751 -> [w762]
                      tunnel: [w762] -> w750
                      tunnel: w749 -> [w761]
                      tunnel: w752 -> [w767]
                      tunnel: w750 -> [w766]
                      tunnel: [w764] -> w744
                      frame #0 {
                        n485 = call-poly <vilib>:"DAQmx Write.vi"("task/channels in"=w757, "data"=TRUE, "error in"=w755) -> ("task out"=w759:refnum<k21>, "error out"=w758:errorcluster)  [unwired: 10 in, 1 out]
                      }
                      frame #1 {
                        n486 = Wait Until Next ms Multiple(millisecond multiple=w761) -> ()  [unwired: 1 out]
                      }
                      frame #2 {
                        n487 = call-poly <vilib>:"DAQmx Write.vi"("task/channels in"=w767, "data"=FALSE, "error in"=w766) -> ("error out"=w764:errorcluster)  [unwired: 10 in, 2 out]
                      }
                    }
                    n488 = Bundle By Name(cluster=w746, "error out"=w744) -> (w745:T13)
                  }
                }
              }
              event "Block laser beam": Value Change {
                n489 = event-data() -> ("NewVal"=w768:bool)  [unwired: 1 in, 5 out]
                n490 = flat-sequence {
                  tunnel: w770 -> [w778]
                  tunnel: w770 -> [w775]
                  tunnel: [w774] -> w769
                  tunnel: w768 -> [w773]
                  frame #0 {
                    n491 = Unbundle By Name(w778) -> ("error out"=w777:errorcluster, "Laser shutter task"=w771:refnum<k21>)
                    n492 = Not(x=w773) -> (.not. x?=w772:bool)
                    n493 = call-poly <vilib>:"DAQmx Write.vi"("task/channels in"=w771, "data"=w772, "error in"=w777) -> ("error out"=w776:errorcluster)  [unwired: 10 in, 2 out]
                    n494 = Bundle By Name(cluster=w775, "error out"=w776) -> (w774:T13)
                  }
                }
              }
              event "Clean": Value Change {
                n495 = event-data() -> ("NewVal"=w782:bool)  [unwired: 1 in, 5 out]
                n496 = case shown="Vrai" w782 {
                  tunnel: w781 -> [w783 w784]
                  tunnel: [w783 w791] -> w780
                  tunnel: w779 -> [_ w790]
                  frame False {
                  }
                  frame True {
                    n497 = control-ref of="Kinetics"() -> (w786:refnum<vi>)
                    n498 = property on="mimic main cursor move" class="Bool (strict)"() -> ("Value"=w789:bool)  [unwired: 2 in, 2 out]
                    n499 = call "clean-change-cursor-kin-event.vi"("cluster in"=w784, "Kinetics graph"=w786) -> ("cluster out"=w785:T13)
                    n500 = Not(x=w789) -> (.not. x?=w788:bool)
                    n501 = Unbundle By Name(w790) -> ("Update graphs of exp"=w787:refnum<user-event>)
                    n502 = property on="mimic main cursor move" class="Bool (strict)"("Val(Sgnl)"=w788) -> ()  [unwired: 2 in, 2 out]
                    n503 = call "clean-expSD.vi"("Update graphs of exp"=w787, "input cluster"=w785) -> ("output cluster"=w791:T13)
                  }
                }
              }
              event "LogY": Value Change {
                n504 = event-data() -> ("NewVal"=w794:bool)  [unwired: 1 in, 5 out]
                n505 = Boolean To (0,1)(Boolean=w794) -> (0, 1=w793:i16)
                n506 = property on="Kinetics" class="GraphXY (strict)"("YScale.Mapping Mode"=w793) -> ()  [unwired: 2 in, 2 out]
              }
              event "clean mode": Value Change {
                n507 = event-data() -> ("NewVal"=w795:enum32{"delete", "approximate"})  [unwired: 1 in, 5 out]
                n508 = global write "globalVarSD.vi" "clean mode"(w795) -> ()
              }
              event "sigma": Value Change {
                n509 = event-data() -> ("NewVal"=w798:dbl)  [unwired: 1 in, 5 out]
                n510 = global write "globalVarSD.vi" "sigma"(w798) -> ()
              }
              event Menu Selection (User) {
                n511 = event-data() -> ("ItemTag"=w800:string)  [unwired: 1 in, 6 out]
                n512 = case shown="\"Quit\"" w800 {
                  tunnel: w801 -> [_ w807]
                  tunnel: [FALSE ("Cell in place") w804] -> w799
                  frame "Faux", Default {
                  }
                  frame "Quit" {
                    n513 = Unbundle By Name(w807) -> ("Stop event"=w805:refnum<user-event>)
                    n514 = call "stop-eventSD.vi"("Stop Event in"=w805) -> (1:"Cell in place"=w804:bool, 2:"Cell in place"=w806:bool)
                    n515 = property on="Cell in place" class="Bool (strict)"("Value"=w806) -> ()  [unwired: 2 in, 2 out]
                  }
                }
              }
              event "wavelength fix": Value Change {
                n516 = event-data() -> ("NewVal"=w809:dbl)  [unwired: 1 in, 5 out]
                n517 = flat-sequence {
                  tunnel: w809 -> [w812]
                  frame #0 {
                    n518 = call "verify-selected-wavesSD.vi"("in wave"=w812) -> ("closet wave"=w810:dbl, "closest index"=w811:i32)  [unwired: 1 in, 2 out]
                    n519 = global write "globalVarSD.vi" "wavelength fix index"(w811) -> ()
                    n520 = local write "wavelength fix"(w810) -> ()
                  }
                }
              }
              event "Break measurement": Value Change {
                n521 = event-data() -> ("NewVal"=w814:bool)  [unwired: 1 in, 5 out]
                n522 = case shown="Vrai" w814 {
                  selector: w814 -> [_ w815]
                  frame False {
                  }
                  frame True {
                    n523 = global write "globalVarSD.vi" "Break measurement"(w815) -> ()
                  }
                }
              }
              event "Relay key": Value Change {
                n524 = event-data() -> ("NewVal"=w818:bool)  [unwired: 1 in, 5 out]
                n525 = flat-sequence {
                  tunnel: w819 -> [w824]
                  tunnel: w818 -> [w825]
                  tunnel: [w822] -> w816
                  tunnel: w817 -> [w820]
                  frame #0 {
                    n526 = Unbundle By Name(w824) -> ("Relay key task"=w826:refnum<k21>)
                    n527 = Unbundle By Name(w820) -> ("error out"=w821:errorcluster)
                    n528 = call-poly <vilib>:"DAQmx Write.vi"("task/channels in"=w826, "data"=w825, "error in"=w821) -> ("error out"=w823:errorcluster)  [unwired: 10 in, 2 out]
                    n529 = Bundle By Name(cluster=w820, "error out"=w823) -> (w822:T13)
                  }
                }
              }
              event "accuracy": Value Change {
                n530 = event-data() -> ("NewVal"=w828:string)  [unwired: 1 in, 5 out]
                n531 = global write "globalVarSD.vi" "accuracy"(w828) -> ()
              }
            }
            n532 = Unbundle By Name(w267) -> ("error out"=w266:errorcluster)
            n533 = call <vilib>:"Simple Error Handler.vi"("error in (no error)"=w266) -> ()  [unwired: 4 in, 5 out]
          }
          n534 = while "Protection Loop" {
            tunnel: w104 -> [w137]
            shift-right: [w129] -> w110
            shift-left: w117 -> [w131]
            tunnel: [w130] -> w111
            stop <- w135 stop-if-true
            n535 = Unbundle By Name(w137) -> ("Protection"=w136:refnum<event-registration>, "Faraday Cup task"=w133:refnum<k21>, "Accelerator task"=w132:refnum<k21>, "heater Alarm task"=w128:refnum<k21>, "Motor task"=w127:refnum<k21>, "Relay key task"=w126:refnum<k21>)
            n536 = event shown="[0] Timeout" {
              selector: w136 -> [_ _]
              dyn-events: [_ _] -> w130
              timeout: 1000 -> [_ _]
              tunnel: [_ w205] -> w135
              tunnel: w133 -> [w144 w204]
              tunnel: w132 -> [w143 w203]
              tunnel: [w141 w187] -> w129
              tunnel: w131 -> [w142 w184]
              tunnel: w128 -> [w139 w202]
              tunnel: w127 -> [_ w194]
              tunnel: w126 -> [w138 w182]
              event Timeout {
                n537 = event-data() -> ()  [unwired: 1 in, 3 out]
                n538 = global read "globalVarSD.vi" "Dev"() -> (w140:bool)
                n539 = case shown="Faux" w140 {
                  tunnel: w144 -> [w170 _]
                  tunnel: w143 -> [w169 _]
                  tunnel: w142 -> [w161 w179]
                  tunnel: [w154 w179] -> w141
                  tunnel: w139 -> [w162 _]
                  tunnel: w138 -> [w145 _]
                  frame False {
                    n540 = call-poly <vilib>:"DAQmx Read.vi"("task/channels in"=w170, "error in"=w161) -> ("data"=w167:bool, "error out"=w168:errorcluster)  [unwired: 11 in, 1 out]
                    n541 = Not(x=w167) -> (.not. x?=w164:bool)
                    n542 = call-poly <vilib>:"DAQmx Read.vi"("task/channels in"=w162, "number of samples per channel"=1000, "error in"=w161) -> ("data"=w159:dbl[], "error out"=w153:errorcluster)  [unwired: 10 in, 1 out]
                    n543 = call-poly <vilib>:"Mean.vi"("X"=w159) -> ("mean"=w158:dbl)  [unwired: 1 out]
                    n544 = Not(x="Block accelerator") -> (.not. x?=w165:bool)
                    n545 = Or(x=w164, y=w165) -> (x .or. y?=w163:bool)
                    "Accelerator" <- w163
                    n546 = Multiply(x=w158, y=1000000.0) -> (x*y=w150:dbl)
                    "Alarm current" <- w150
                    n547 = Greater?(x=w150, y="current Alarm, uA") -> (0:w148:bool)
                    n548 = Less?(x=w150, y="current Alarm break, uA") -> (x < y?=w146:bool)
                    n549 = call-poly <vilib>:"DAQmx Write.vi"("task/channels in"=w169, "data"=w163, "error in"=w168) -> ("error out"=w156:errorcluster)  [unwired: 10 in, 2 out]
                    n550 = Or(x=w148, y=w146) -> (x .or. y?=w147:bool)
                    "ALARM" <- w147
                    n551 = property on="ALARM" class="Bool (strict)"("Blinking"=w147) -> ()  [unwired: 2 in, 2 out]
                    n552 = case shown="Vrai" w147 {
                      tunnel: w153 -> [w171 w176]
                      tunnel: [w171 w177] -> w152
                      tunnel: w145 -> [_ w175]
                      frame False {
                      }
                      frame True {
                        n553 = call-poly <vilib>:"DAQmx Write.vi"("task/channels in"=w175, "data"=FALSE, "error in"=w176) -> ("error out"=w173:errorcluster)  [unwired: 10 in, 2 out]
                        n554 = invoke on="Relay key" class="Bool (strict)" method="RétablirValParDéfaut"(error in=w173) -> (error out=w172:errorcluster)  [unwired: 2 in, 2 out]
                        n555 = call <vilib>:"Play Sound File.vi"("error in (no error)"=w172, "path"="path alarm sound") -> ("error out"=w177:errorcluster)  [unwired: 8 in, 1 out]
                      }
                    }
                    n556 = Build Array(w156, w152) -> (w155:errorcluster[])
                    n557 = Merge Errors(w155) -> (w154:errorcluster)
                  }
                  frame True {
                  }
                }
              }
              event User Event {
                n558 = event-data() -> ("Stop"=w205:bool)  [unwired: 1 in, 4 out]
                n559 = call-poly <vilib>:"DAQmx Write.vi"("task/channels in"=w182, "data"=FALSE) -> ("task out"=w181:refnum<k21>)  [unwired: 11 in, 2 out]
                n560 = call <vilib>:"DAQmx Stop Task.vi"("task/channels in"=w194, "error in"=w184) -> ("task out"=w196:refnum<k21>, "error out"=w195:errorcluster)  [unwired: 12 in]
                n561 = call <vilib>:"DAQmx Stop Task.vi"("task/channels in"=w204, "error in"=w184) -> ("task out"=w197:refnum<k21>, "error out"=w201:errorcluster)  [unwired: 12 in]
                n562 = call <vilib>:"DAQmx Stop Task.vi"("task/channels in"=w203, "error in"=w184) -> ("task out"=w198:refnum<k21>, "error out"=w193:errorcluster)  [unwired: 12 in]
                n563 = call <vilib>:"DAQmx Stop Task.vi"("task/channels in"=w202, "error in"=w184) -> ("task out"=w199:refnum<k21>, "error out"=w200:errorcluster)  [unwired: 12 in]
                n564 = call <vilib>:"DAQmx Stop Task.vi"("task/channels in"=w181, "error in"=w184) -> ("task out"=w185:refnum<k21>, "error out"=w186:errorcluster)  [unwired: 12 in]
                n565 = call <vilib>:"DAQmx Clear Task.vi"("task in"=w196, "error in"=w195) -> ("error out"=w192:errorcluster)  [unwired: 13 in]
                n566 = call <vilib>:"DAQmx Clear Task.vi"("task in"=w197, "error in"=w201) -> ("error out"=w191:errorcluster)  [unwired: 13 in]
                n567 = call <vilib>:"DAQmx Clear Task.vi"("task in"=w198, "error in"=w193) -> ("error out"=w190:errorcluster)  [unwired: 13 in]
                n568 = call <vilib>:"DAQmx Clear Task.vi"("task in"=w199, "error in"=w200) -> ("error out"=w189:errorcluster)  [unwired: 13 in]
                n569 = call <vilib>:"DAQmx Clear Task.vi"("task in"=w185, "error in"=w186) -> ("error out"=w183:errorcluster)  [unwired: 13 in]
                n570 = Build Array(w192, w191, w190, w189, w183) -> (w188:errorcluster[])
                n571 = Merge Errors(w188) -> (w187:errorcluster)
              }
            }
            n572 = call <vilib>:"Simple Error Handler.vi"("error in (no error)"=w129) -> ()  [unwired: 4 in, 5 out]
          }
          n573 = Unbundle By Name(w122) -> ("error out"=w109:errorcluster, "Laser shutter task"=w116:refnum<k21>, "Accelerator task"=w113:refnum<k21>, "Motor task"=w112:refnum<k21>)
          n574 = Unregister For Events(event registration refnum=w124, error in=w109) -> (error out=w108:errorcluster)
          n575 = call <vilib>:"DAQmx Clear Task.vi"("task in"=w116, "error in"=w108) -> ("error out"=w115:errorcluster)  [unwired: 13 in]
          n576 = Unregister For Events(event registration refnum=w111, error in=w110) -> (error out=w106:errorcluster)
          n577 = call <vilib>:"DAQmx Clear Task.vi"("task in"=w113, "error in"=w115) -> ("error out"=w114:errorcluster)  [unwired: 13 in]
          n578 = Unregister For Events(event registration refnum=w123, error in=w105) -> (error out=w120:errorcluster)
          n579 = call <vilib>:"DAQmx Clear Task.vi"("task in"=w112, "error in"=w114) -> ("error out"=w107:errorcluster)  [unwired: 13 in]
          n580 = Build Array(w120, w107, w106) -> (w119:errorcluster[])
          n581 = Merge Errors(w119) -> (→"error out":errorcluster)
        }
      }
    }
  }
